vi "Core_Chem_User_Interface_v1.2.vi"() -> ()   [LabVIEW 2014]
uses:
  C:/Program Files (x86)/National Instruments/LabVIEW 2014/examples/Data Communication/Network Streams/Simple Network Streams/support/Network Stream Command.ctl
  <vilib>/dex/Stream Element Allocation Mode.ctl
  <vilib>/Platform/TimedLoop/XDataNode/timing_clust.ctl
  <vilib>/Platform/TimedLoop/XDataNode/nitl_modes.ctl
  <vilib>/Platform/TimedLoop/XDataNode/wakeup.ctl
  <vilib>/Utility/tcp.llb/UDP Multicast Read-Only Open.vi
  <vilib>/platform/TimedLoop/XDataNode/XDataNode.xnode
  <vilib>/Platform/TimedLoop/XDataNode/XDNodeRunTimeDep.lvlib
  <vilib>/FTP/NI_FTP.lvlib
panel:
  out "Create folder error out 2":errorcluster
  out "Network to cRIO live status":bool
  out "Create folder error out":errorcluster
  in  "Confirm Flight Number":bool
  out "PRTAFT_UDP_In":string
  out "TWBOZO01":string
  out "CABOZO01":string
  out "TEIOZO01":string
  out "CHTSOO01":string
  out "CHFGGA01":string
  out "AL52CO01":string
  in  "Flight Number":string
  in  "Tab Control":T1(tab)
  out "PRTAFT_DLU":string
  out "MFM":dbl(graph)
  in  "name":string="239.1.4.6"
  in  "Port":u16=50001
  out "FGGA":string
  out "CO":string
  out "Ozone":string
  out "Cabin Ozone":string
  out "Ambient Ozone":string
  out "SO2":string
  out "Raw Signal":dbl(graph)
  out "CO Concentration":dbl(graph)
  out "Fluorsecence Cell Pressure":dbl(graph)
  out "Monochromater Flow":dbl(graph)
  out "Lamp Flow Controller":dbl(graph)
  in  "CO UDP Time Offset":i32=1
  out "CO2 Pressure\nDelivery (PSIA)":dbl(slide) scale=0.0..100.0
  out "CO CAL Status":bool
  out "Std\nContent (barG)":dbl(slide) scale=0.0..220.0
  out "N2\nContent (barG)":dbl(slide) scale=0.0..220.0
  out "CO2\nContent (barG)":dbl(slide) scale=0.0..170.0
  in  "CO CAL":bool
  in  "CO Vacuum (eV7)":bool
  out "CO Event error out":errorcluster
  out "CO command sender error out":errorcluster
  out "CO Zero":T2(array[cluster])
  out "CO Sensitivity":T3(array[cluster])
  in  "Ozone eV6":bool
  out "TEI49C Sample Flow B":dbl(graph)
  out "TEi49C Concentration":dbl(graph)
  out "TEI49C Sample Flow A":dbl(graph)
  out "Ozone Event error out":errorcluster
  out "Ozone command sender error out":errorcluster
  out "Ozone Zeroing\nTime Remain (sec)":u32
  in  "Ozone Zeroing":bool
  in  "Ozone UDP Time Offset":i32=1
  in  "FGGA Pump":bool
  in  "FGGA Shutdown":bool
  in  "eV1":bool
  in  "eV2":bool
  in  "MFC_1\nSLPM Value":dbl
  in  "eV3":bool
  in  "eV4":bool
  in  "FGGA Restart":bool
  out "MFC1 Cal Flow":dbl(graph)
  out "Cell temperature":dbl(graph)
  out "Cell pressure":dbl(graph)
  out "CO2 Dry":dbl(graph)
  out "CH4 Dry":dbl(graph)
  out "H2O":dbl(graph)
  out "CO2":dbl(graph)
  out "CH4":dbl(graph)
  in  "Flush High Tank":bool
  in  "Flush Low Tank":bool
  in  "Flush Target Tank":bool
  out "Flush High Tank\nTime Remain (sec)":u32
  out "Flush Low Tank\nTime Remain (sec)":u32
  out "Flush Target Tank\nTime Remain (sec)":u32
  in  "High Cal":bool
  out "High Cal\nFlush Time Remain (sec)":u32
  out "High Cal\nCal Time Remain (sec)":u32
  in  "Low Cal":bool
  in  "Target Cal":bool
  in  "Span Cal":bool
  out "Low Cal\nFlush Time Remain (sec)":u32
  out "Low Cal\nCal Time Remain (sec)":u32
  out "Target Cal\nFlush Time Remain (sec)":u32
  out "Target Cal\nCal Time Remain (sec)":u32
  in  "MFC_1 User Set Value":dbl=3.0
  out "FGGA command sender error out":errorcluster
  out "FGGA Event Error out":errorcluster
  in  "FGGA UDP Time Offset":i32=1
  in  "FGGA pump\nsync to WoW":bool
  out "WoW Flag":string="0"
  in  "Inst_alm_thresh":i32=220
  in  "3hr_alm_thresh":i32=80
  in  "Simulate Inst Conc":i32
  in  "Simulate 3hr Average Conc":dbl
  in  "Simulate 2B Conc":bool
  out "2B Ozone concentration":dbl(graph)
  out "2B Ozone flow rate":dbl(graph)
  out "2BOzone Event error out":errorcluster
  out "2BOzone command sender error out":errorcluster
  in  "Ambient = OFF\nCabin = ON":bool
  in  "eV9 Flush User\nset time (sec)":i32=15
  in  "eV9 flush User\nset time (sec)":i32=60
  in  "eV8 User\nset time (sec)":i32=120
  in  "eV9":bool
  in  "eV8":bool
  in  "SO2 eV6":bool
  in  "MFC_2\nSLPM Value":dbl
  in  "MFC_3\nSLPM Value":dbl=2.0
  in  "Simulate STEL Conc":dbl
  in  "Simulate TWA Conc":dbl
  in  "SO2 Offset":dbl
  in  "SO2 Slope":dbl=1.0
  in  "10mins STEL Limit":i32=700
  in  "8hr TWA Limit":i32=490
  in  "Simulate Conc":bool
  out "TEI43i MFC2 Cal Flow":dbl(graph)
  out "TEI43i MFC3 Sample Flow":dbl(graph)
  out "TEi43C Concentration":dbl(graph)
  out "TEI43C Sample Flow":dbl(graph)
  out "SO2 Event error out":errorcluster
  out "SO2 command sender error out":errorcluster
  in  "SO2 Flush":bool
  in  "SO2 CAL":bool
  in  "MFC_2 User Set Value":dbl=2.5
  in  "MFC_3 User Set Value":dbl=2.0
  out "SO2 Flush\nTime Remain (sec)":u32
  in  "SO2 Zeroing":bool
  out "SO2 Zeroing\nTime Remain (sec)":u32
  out "SO2 CAL\nTime Remain (sec)":u32
  in  "SO2 UDP Time Offset":i32=1
  in  "cRIO File IO Stop\n(USB Flash Drive Unmount)":bool
  in  "FTP ASCII Files to Local":bool
  in  "Transfer FGGA Files":bool
  out "File List":string[](array[string])
  out "FGGA File Transfer Error out":errorcluster
  out "Move to FM Error out":errorcluster
  out "USB Disk Space Used %":dbl(slide) scale=0.0..100.0
  out "PTP Sync":bool
  out "CPU Total %":dbl(graph)
  # "ch4\nco2\nh2o\npress_torr\ntemp_c\nfit_flag\nrda_usec\nrdb_usec\nch4_dry\nco2_dry\nMFC_1_absolute_pressure\nMFC_1_temperature\nMFC_1volumetic_flow\nMFC_1mass_flow\nMFC_1set_point\nV1\nV2\nV3\nV4\nrestart_FGGA\nFGGA_Pump\nCAL_MFC_1Set_Value"
  # "conc\ntemp\npress\nflow\nthreehr_oz\nInst_alarm\nthreehr_alarm"
  # "conc\ntemp\npress\nflow"
  # "concentration\npmt_volt\nlamp_volt\nlamp_intens\ninternal_temper\nreact_temper\nreact_press\nflow\nflags\nten_min_so2\neight_hr_so2\nten_min_so2_alm\neight_hr_so2_alm\nMFC_2absolute_pressure\nMFC_2temperature\nMFC_2volumetic_flow\nMFC_2mass_flow\nMFC_2set_point\nMFC_3_absolute_pressure\nMFC_3_temperature\nMFC_3volumetic_flow\nMFC_3mass_flow\nMFC_3set_point\nV6\nV8\nV9\nMFC2_Set_Value\nMFC3_Set_Value"
  # "conc\nbenchtemp\npress\ncellAint\ncellBint\nFlowA\nFlowB\nlamptemp\nflag\nV6"
  # "conc\ncounts\nsens\nzero\nlampflow\nlamptemp\nmonoflow\nmonotemp\nmonopress\ncellpress\ncalpress\ntemppmt\ncalconc\nerr\ncal_counter\nerr_counter\nCO_vacuum_status\nIn_Cal\nALEG1_press_delivery\nALREG1_press_content\nALREG2_press_content\nALREG3_press_content"
  # "DIRECT CONTROL"
  # "DIRECT CONTROLS"
  # "DIRECT CONTROLS"
  # "TEi43c"
  # "TEi43i"
  # "SO2 FLUSH SETTING"
  # "SO2 CAL SETTINGS"
  # "DIRECT CONTROLS"
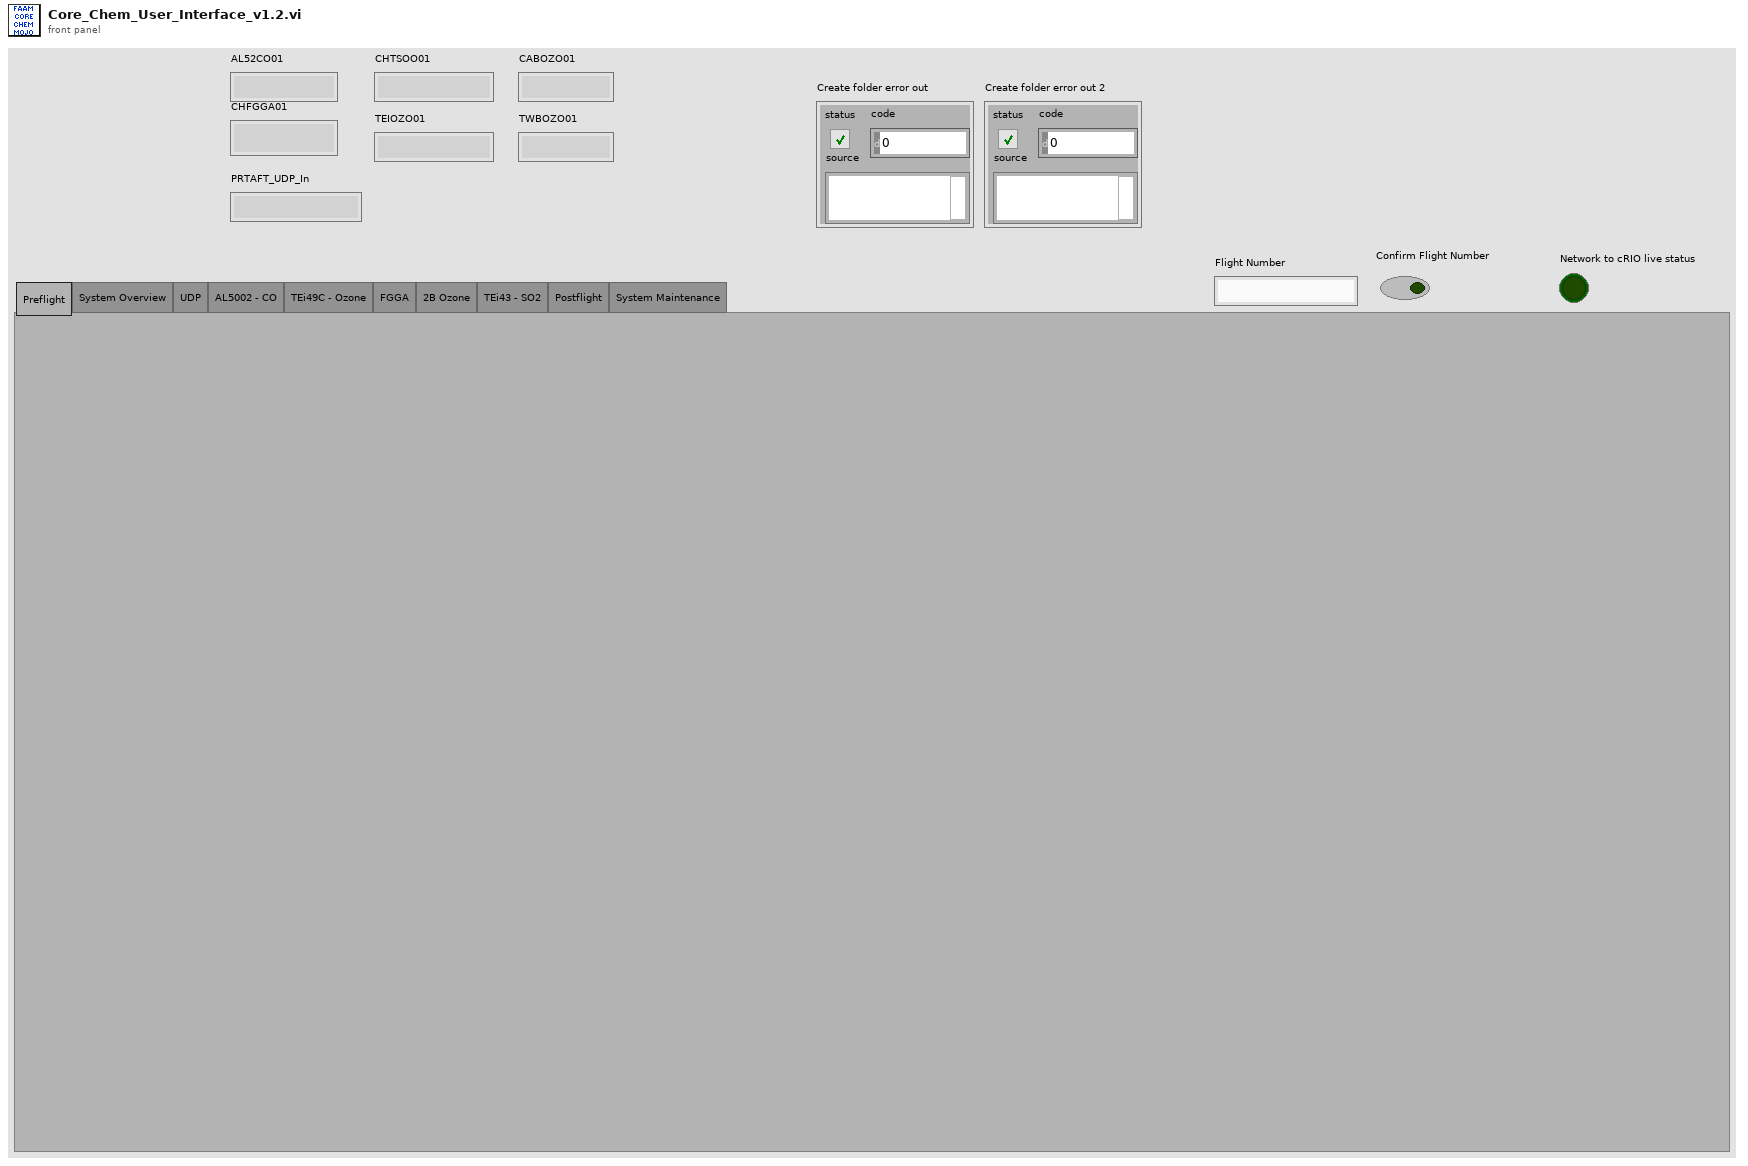
[diagram p1: front panel]
types:
  T1 = enum32{"Preflight", "System Overview", "UDP", "AL5002 - CO", "TEi49C - Ozone", "FGGA", "2B Ozone", "TEi43 - SO2", "Postflight", "System Maintenance"}
  T2 = cluster{"time stamp":timestamp, "CO Offset":dbl}[]
  T3 = cluster{"time stamp":timestamp, "CO Sensitivity":dbl}[]
  T4 = typedef "Network Stream Command.ctl" = cluster{"Message":string, "Message Data":variant}
  T5 = typedef "Stream Element Allocation Mode.ctl" = u32
  T6 = typedef "XDNodeRunTimeDep.lvlib/timing_clust.ctl" = cluster{"Expected End [f-1]":u64, "Actual End [f-1]":u64, "Finished Late? [f-1]":bool, "Expected End [i-1]":u64, "Actual End [i-1]":u64, "Finished Late? [i-1]":bool, "Expected Start [i]":u64, "Actual Start [i]":u64, "Expected Start [f]":u64, "Actual Start [f]":u64, "Source Name":string, "Structure Name":string, "Period":i64, "Deadline":i64, "Offset":i64, "Start":i64, "Priority":i32, "Timeout":i32, "Mode":T7, "Wakeup Reason":T8, "Error":errorcluster, "Source Type":string, "Secondary Source Type":string, "Global End Time":u64, "Global Start Time":u64, "Frame Duration":u64, "Iteration Duration":u64, "Assigned CPU":i32, "I/O Scan Engine Mode":u32}
  T7 = typedef "XDNodeRunTimeDep.lvlib/nitl_modes.ctl" = enum32{"No Change", "Process missed periods, maintain original phase", "Discard missed periods, maintain original phase", "Process missed periods, ignore original phase", "Discard missed periods, ignore original phase"}
  T8 = typedef "XDNodeRunTimeDep.lvlib/wakeup.ctl" = enum32{"Normal", "Aborted", "Asynchronous wakeup", "Timing source error", "Timed loop error", "Timeout"}
  T9 = typedef "NI_FTP.lvlib/FTP Session.ctl" = refnum<k5>
  T10 = typedef "NI_FTP.lvlib/FTP File Info.ctl" = cluster{"type":enum16{"unknown", "file", "dir", "link"}, "permissions":string, "owner":string, "group":string, "size":i32, "date":string, "name":string, "link name":string}
  T11 = cluster{"Message":string, "Message 2":string, "Message 3":string}
  T12 = cluster{"Message":string, "Message 2":string, "Message 3":string, "Message 4":string}
  T13 = cluster{"Message":string, "Message 3":string, "Message 4":string}
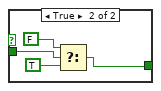
[diagram p8: hidden frame]
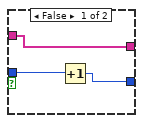
[diagram p13: hidden frame]
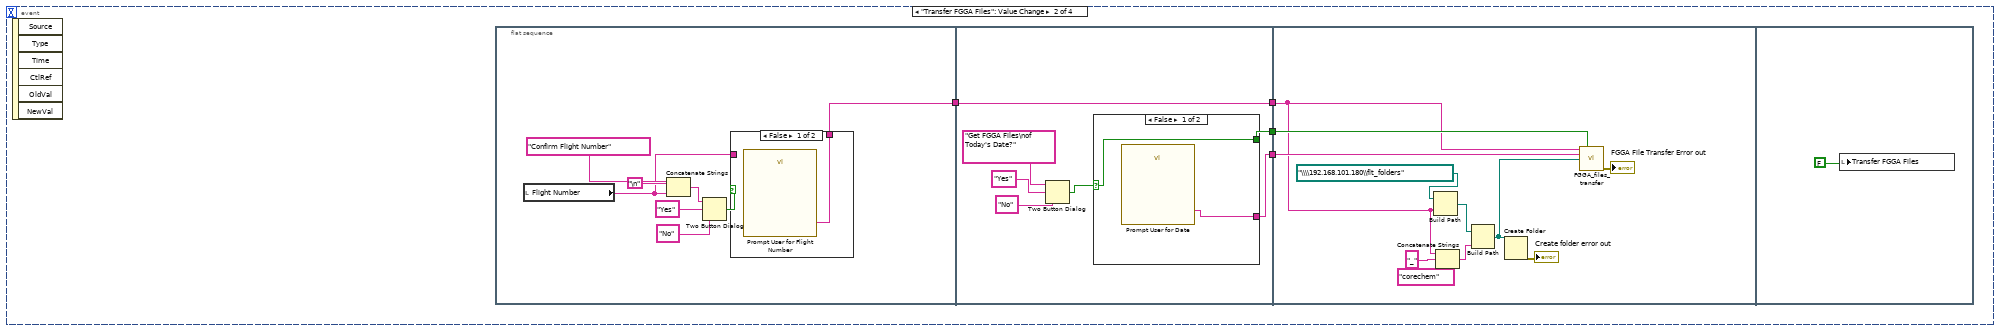
[diagram p15: hidden frame]
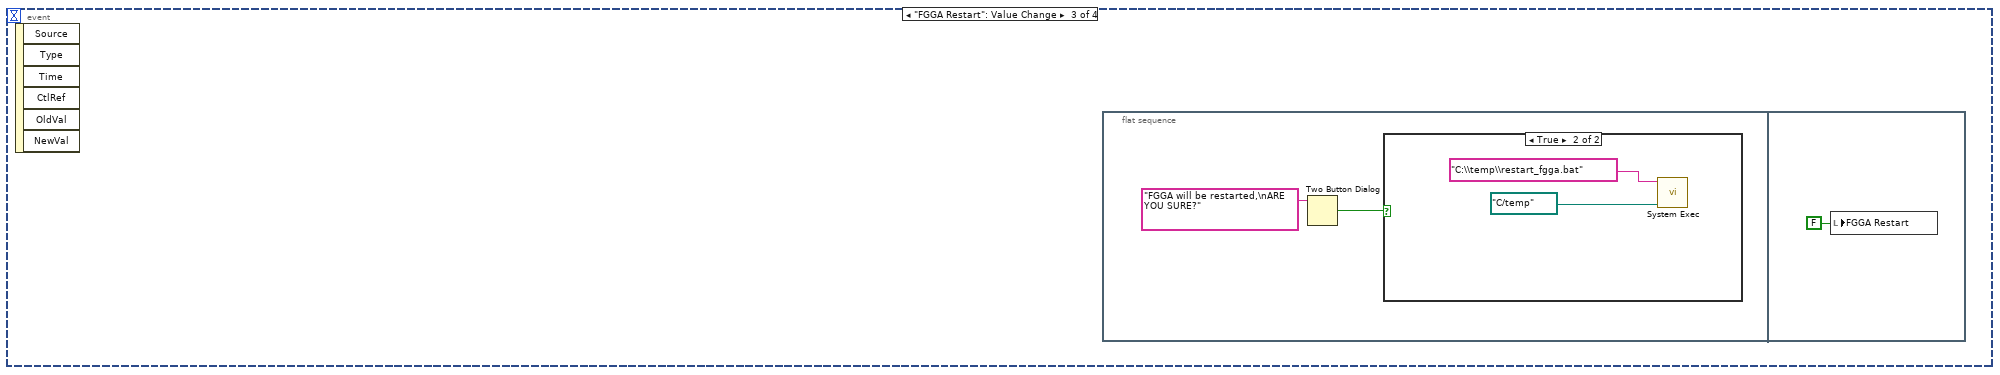
[diagram p18: hidden frame]
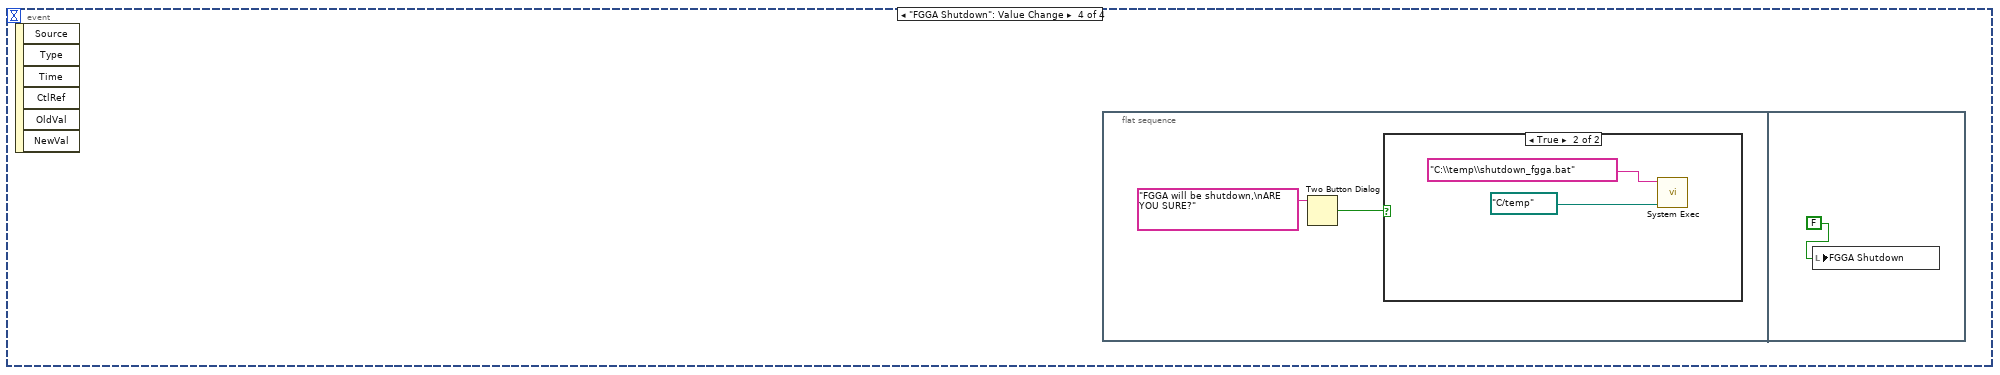
[diagram p20: hidden frame]
diagram:
  w4 = "XXXX"
  w7 = 0
  w8 = 0.0
  w14 = T4 {"Message"="", "Message Data"=variant} ("Message Cluster")
  w20 = T5 0 items=["allocate as needed", "pre-allocate"] ("element allocation mode")
  w26 = T4 {"Message"="", "Message Data"=variant} ("Message Cluster")
  w32 = T5 0 items=["allocate as needed", "pre-allocate"] ("element allocation mode")
  w37 = T4 {"Message"="", "Message Data"=variant} ("Message Cluster")
  w43 = T5 0 items=["allocate as needed", "pre-allocate"] ("element allocation mode")
  w53 = T5 0 items=["allocate as needed", "pre-allocate"] ("element allocation mode")
  w55 = T4 {"Message"="", "Message Data"=variant} ("Message Cluster")
  w62 = T5 0 items=["allocate as needed", "pre-allocate"] ("element allocation mode")
  w64 = T4 {"Message"="", "Message Data"=variant} ("Message Cluster")
  n1 = local write "cRIO File IO Stop\n(USB Flash Drive Unmount)"(FALSE ("Stop File Write")) -> ()
  n2 = local write "Flight Number"(w4) -> ()
  n3 = while {
    shift-right: [w68] -> _
    shift-left: w4 -> [w67]
    stop <- FALSE stop-if-true
    n4 = Not Equal?(x=w67, y="Flight Number") -> (x != y?=w70:bool)
    n5 = case shown="True" w70 {
      tunnel: [w73 w74] -> w68
      tunnel: "Flight Number" -> [_ w74]
      tunnel: w67 -> [w73 _]
      frame False {
      }
      frame True {
        n6 = One Button Dialog(message="Flight Number changed,\nPress flight number button to confirm") -> ()  [unwired: 1 in, 1 out]
      }
    }
    n7 = Wait (ms)(milliseconds to wait=u32 1000) -> ()  [unwired: 1 out]
  }
  n8 = while {
    stop <- FALSE stop-if-true
    # "UDP Read"
    n9 = String To IP(1:"name") -> (0:w81:u32)
    n10 = call-poly <vilib>:"UDP Multicast Open.vi"("multicast addr"=w81, "port"="Port") -> ("error out"=w79:errorcluster, "connection ID"=w78:refnum<k16>)  [unwired: 7 in, 1 out]
    n11 = Wait (ms)(milliseconds to wait=u32 1000) -> ()  [unwired: 1 out]
    n12 = case shown="No Error" w79 {
      selector: w79 -> [w85 _]
      tunnel: w78 -> [w84 _]
      frame No Error {
        w83 = ""
        n13 = while {
          tunnel: w85 -> [w131]
          tunnel: w84 -> [w130]
          shift-right: [w126] -> _
          shift-left: w83 -> [w127]
          shift-right: [w117] -> _
          shift-left: w83 -> [w119]
          shift-right: [w111] -> _
          shift-left: w83 -> [w113]
          shift-right: [w105] -> _
          shift-left: w83 -> [w106]
          shift-right: [w99] -> _
          shift-left: w83 -> [w100]
          shift-right: [w93] -> _
          shift-left: w83 -> [w94]
          shift-right: [w87] -> _
          shift-left: w83 -> [w88]
          stop <- w129 stop-if-true
          n14 = UDP Read(connection ID=w130, 8:w131) -> (data out=w86:string, error out=w129:errorcluster)  [unwired: 2 in, 3 out]
          n15 = Match Pattern(string=w86, regular expression="$TEIOZO01,") -> (match substring=w125:string, after substring=w124:string)  [unwired: 1 in, 2 out]
          n16 = Match Pattern(string=w86, regular expression="$TWBOZO01,") -> (match substring=w103:string, after substring=w102:string)  [unwired: 1 in, 2 out]
          n17 = Match Pattern(string=w86, regular expression="$CABOZO01,") -> (match substring=w109:string, after substring=w108:string)  [unwired: 1 in, 2 out]
          n18 = Match Pattern(string=w86, regular expression="$CHTSOO01,") -> (match substring=w97:string, after substring=w96:string)  [unwired: 1 in, 2 out]
          n19 = Match Pattern(string=w86, regular expression="$CHFGGA01,") -> (match substring=w121:string, after substring=w120:string)  [unwired: 1 in, 2 out]
          n20 = Match Pattern(string=w86, regular expression="$AL52CO01,") -> (match substring=w115:string, after substring=w114:string)  [unwired: 1 in, 2 out]
          n21 = Match Pattern(string=w86, regular expression="$PRTAFT01,") -> (match substring=w92:string, after substring=w91:string)  [unwired: 1 in, 2 out]
          n22 = Concatenate Strings(w125, w124) -> (w123:string)
          n23 = Concatenate Strings(w103, w102) -> (w101:string)
          n24 = Concatenate Strings(w109, w108) -> (w107:string)
          n25 = Concatenate Strings(w97, w96) -> (w95:string)
          n26 = Concatenate Strings(w121, w120) -> (w118:string)
          n27 = Concatenate Strings(w115, w114) -> (w112:string)
          n28 = Concatenate Strings(w92, w91) -> (w89:string)
          n29 = Replace Substring(4:w101, 5:w100) -> (1:w99:string)  [unwired: 2 in, 1 out]
          "TWBOZO01" <- w99
          n30 = Replace Substring(4:w123, 5:w127) -> (1:w126:string)  [unwired: 2 in, 1 out]
          "TEIOZO01" <- w126
          n31 = Replace Substring(4:w107, 5:w106) -> (1:w105:string)  [unwired: 2 in, 1 out]
          "CABOZO01" <- w105
          n32 = Replace Substring(4:w95, 5:w94) -> (1:w93:string)  [unwired: 2 in, 1 out]
          "CHTSOO01" <- w93
          n33 = Replace Substring(4:w112, 5:w113) -> (1:w111:string)  [unwired: 2 in, 1 out]
          "AL52CO01" <- w111
          n34 = Replace Substring(4:w118, 5:w119) -> (1:w117:string)  [unwired: 2 in, 1 out]
          "CHFGGA01" <- w117
          n35 = Replace Substring(4:w89, 5:w88) -> (1:w87:string)  [unwired: 2 in, 1 out]
          "PRTAFT_UDP_In" <- w87
        }
      }
      frame Error {
      }
    }
  }
  n36 = Obtain Queue(name (unnamed)="CO_Command", element data type=w64) -> (queue out=w13:refnum<queue>, error out=w58:errorcluster)  [unwired: 3 in, 1 out]
  n37 = Create Network Stream Writer Endpoint(6:w62, 7:10 ("writer buffer size"), 9:w64, 10:"//192.168.101.17/command/reader/CO" ("reader url"), 11:"/command/writer/CO" ("writer name")) -> (0:w61:errorcluster, 3:w60:refnum<k21>)  [unwired: 2 in]
  n38 = while {
    tunnel: w13 -> [w135]
    tunnel: w58 -> [w134]
    tunnel: [w132] -> _
    stop <- FALSE stop-if-true
    # "CO UI Event Handler Loop"
    n39 = event shown="[4] \"Confirm Flight Number\": Value Change" {
      selector: _ -> [_ _ _ _ _]
      dyn-events: _ -> [_ _ _ _ _]
      timeout: _ -> [_ _ _ _ _]
      tunnel: w135 -> [w142 w149 w153 w160 w167]
      tunnel: w134 -> [w141 w148 w152 w159 w166]
      tunnel: [w136 w143 w151 w158 w165] -> w132
      event "CO CAL": Value Change {
        n40 = event-data() -> ("NewVal"=w139:bool)  [unwired: 1 in]
        n41 = Bundle(cluster=T4 {"Message"="", "Message Data"=variant} ("Message Cluster"), "Message"="CO CAL", "Message Data"=w139) -> (w137:T4)
        n42 = Enqueue Element(queue=w142, element=w137, error in (no error)=w141) -> (error out=w136:errorcluster)  [unwired: 1 in, 2 out]
      }
      event "CO UDP Time Offset": Value Change {
        n43 = event-data() -> ("NewVal"=w146:i32)  [unwired: 1 in]
        n44 = Bundle(cluster=T4 {"Message"="", "Message Data"=variant} ("Message Cluster"), "Message"="UDP Time Offset", "Message Data"=w146) -> (w144:T4)
        n45 = Enqueue Element(queue=w149, element=w144, error in (no error)=w148) -> (error out=w143:errorcluster)  [unwired: 1 in, 2 out]
      }
      event "CO Vacuum (eV7)": Value Change {
        n46 = event-data() -> ("NewVal"=w150:bool)  [unwired: 1 in]
        n47 = Bundle(cluster=T4 {"Message"="", "Message Data"=variant} ("Message Cluster"), "Message"="CO Vacuum", "Message Data"=w150) -> (w154:T4)
        n48 = Enqueue Element(queue=w153, element=w154, error in (no error)=w152) -> (error out=w151:errorcluster)  [unwired: 1 in, 2 out]
      }
      event "cRIO File IO Stop\n(USB Flash Drive Unmount)": Value Change {
        n49 = event-data() -> ("NewVal"=w157:bool)  [unwired: 1 in]
        n50 = Bundle(cluster=T4 {"Message"="", "Message Data"=variant} ("Message Cluster"), "Message"="Stop File Write", "Message Data"=w157) -> (w161:T4)
        n51 = Enqueue Element(queue=w160, element=w161, error in (no error)=w159) -> (error out=w158:errorcluster)  [unwired: 1 in, 2 out]
      }
      event "Confirm Flight Number": Value Change {
        n52 = event-data() -> ()  [unwired: 1 in, 1 out]
        n53 = local read "Flight Number"() -> (w164:string)
        n54 = Bundle(cluster=T4 {"Message"="", "Message Data"=variant} ("Message Cluster"), "Message"="Flight Number", "Message Data"=w164) -> (w168:T4)
        n55 = Enqueue Element(queue=w167, element=w168, error in (no error)=w166) -> (error out=w165:errorcluster)  [unwired: 1 in, 2 out]
      }
    }
    "CO Event error out" <- w132
  }
  n56 = while {
    tunnel: w13 -> [w178]
    shift-right: [w173] -> _
    shift-left: w60 -> [w175]
    shift-right: [w171] -> w49
    shift-left: w61 -> [w177]
    tunnel: w58 -> [w172]
    stop <- w171 stop-if-true
    # "CO UI Command Sender"
    n57 = Dequeue Element(queue=w178, error in (no error)=w172) -> (element=w174:T4)  [unwired: 1 in, 3 out]
    n58 = Unbundle By Name(w174) -> ("Message"=w176:string)
    n59 = case shown="\"UDP Time Offset\"" w176 {
      tunnel: w177 -> [w179 w183 w190 w197 w204 w211]
      tunnel: w175 -> [w180 w186 w193 w200 w207 w214]
      tunnel: w174 -> [_ w185 w192 w199 w206 w213]
      tunnel: [w179 w182 w189 w196 w203 w210] -> w171
      tunnel: [w180 w181 w188 w195 w202 w209] -> w173
      frame "False", Default {
      }
      frame "CO CAL" {
        n60 = shared-variable-write(w186, w183, w185) -> (w184:refnum<k21>, w187:errorcluster)  [unwired: 1 in, 1 out]
        n61 = Flush Stream(8:w187, 11:w184) -> (0:w182:errorcluster, 3:w181:refnum<k21>)  [unwired: 2 in, 1 out]
      }
      frame "UDP Time Offset" {
        n62 = shared-variable-write(w193, w190, w192) -> (w191:refnum<k21>, w194:errorcluster)  [unwired: 1 in, 1 out]
        n63 = Flush Stream(8:w194, 11:w191) -> (0:w189:errorcluster, 3:w188:refnum<k21>)  [unwired: 2 in, 1 out]
      }
      frame "Stop File Write" {
        n64 = shared-variable-write(w200, w197, w199) -> (w198:refnum<k21>, w201:errorcluster)  [unwired: 1 in, 1 out]
        n65 = Flush Stream(8:w201, 11:w198) -> (0:w196:errorcluster, 3:w195:refnum<k21>)  [unwired: 2 in, 1 out]
      }
      frame "Flight Number" {
        n66 = shared-variable-write(w207, w204, w206) -> (w205:refnum<k21>, w208:errorcluster)  [unwired: 1 in, 1 out]
        n67 = Flush Stream(8:w208, 11:w205) -> (0:w203:errorcluster, 3:w202:refnum<k21>)  [unwired: 2 in, 1 out]
      }
      frame "CO Vacuum" {
        n68 = shared-variable-write(w214, w211, w213) -> (w212:refnum<k21>, w215:errorcluster)  [unwired: 1 in, 1 out]
        n69 = Flush Stream(8:w215, 11:w212) -> (0:w210:errorcluster, 3:w209:refnum<k21>)  [unwired: 2 in, 1 out]
      }
    }
  }
  "CO command sender error out" <- w49
  n70 = node-c288() -> (w12:T6)  [unwired: 4 in]
  n71 = Initialize Array(cluster{"time stamp":timestamp, "Y":dbl} {"time stamp"=timestamp(0 s since 1904-01-01), "Y"=0.0}, 30 ("dimension size")) -> (w9:cluster{"time stamp":timestamp, "Y":dbl}[])
  n72 = timed-loop {
    timing: w12 -> [_]
    timing-out: [_] -> w11
    stop <- _ stop-if-true
    # "PC Tasks"
    n73 = node-c288() -> ()  [unwired: 1 in, 1 out]
    n74 = event shown="[0] \"FTP ASCII Files to Local\": Value Change" {
      selector: _ -> [_ _ _ _]
      dyn-events: _ -> [_ _ _ _]
      timeout: _ -> [_ _ _ _]
      event "FTP ASCII Files to Local": Value Change {
        n75 = event-data() -> ()  [unwired: 1 in, 1 out]
        n76 = flat-sequence {
          tunnel: [w224] -> w218
          tunnel: [w236] -> w223
          tunnel: [w235] -> w221
          tunnel: [w234] -> w219
          tunnel: w218 -> [w234]
          tunnel: w223 -> [w294]
          tunnel: [w294] -> w222
          tunnel: w221 -> [w290]
          tunnel: [w289] -> w220
          tunnel: w219 -> [w289]
          tunnel: w222 -> [w300]
          tunnel: w220 -> [w295]
          frame #0 {
            n77 = local read "Flight Number"() -> (w226:string)
            n78 = Concatenate Strings("Confirm Flight Number" ("message"), "\n", w226) -> (w230:string)
            n79 = Two Button Dialog(message=w230, 1:"No" ("F button name (\"Cancel\")"), 2:"Yes" ("T button name (\"OK\")")) -> (T button?=w227:bool)
            n80 = case shown="False" w227 {
              tunnel: w226 -> [_ w233]
              tunnel: [w232 w233] -> w224
              frame False {
                n81 = call "Prompt User for Flight Number2"() -> ("Flight Number BXXX"=w232:string)  [unwired: 17 in, 2 out]
              }
              frame True {
              }
            }
          }
          frame #1 {
            n82 = Get Date/Time In Seconds() -> (seconds since 1Jan1904=w240:timestamp)
            n83 = Format Date/Time String(time format string (%c)="%Y%m%d", seconds (now)=w240) -> (date/time string=w238:string)  [unwired: 1 in]
            n84 = call <vilib>:"FTP Open Session.vi"("address"="192.168.101.17") -> ("error out"=w255:errorcluster, "ftp session"=w256:T9)  [unwired: 7 in, 2 out]
            n85 = Concatenate Strings("Use Today's Date" ("message"), "\r", w238) -> (w244:string)
            n86 = call <vilib>:"FTP Logon.vi"("error in (no error)"=w255, "password"="", "user"="anonymous", "ftp session"=w256) -> ("error out"=w252:errorcluster, "ftp session out"=w251:T9)  [unwired: 4 in, 2 out]
            n87 = Two Button Dialog(message=w244, 1:"No" ("F button name (\"Cancel\")"), 2:"Yes" ("T button name (\"OK\")")) -> (T button?=w241:bool)
            n88 = case shown="False" w241 {
              tunnel: [w259 w260] -> w235
              tunnel: w238 -> [_ w260]
              frame False {
                n89 = call "Prompt User for Date"() -> ("Date"=w259:string)  [unwired: 17 in, 2 out]
              }
              frame True {
              }
            }
            n90 = call <vilib>:"FTP Directory Listing.vi"("error in (no error)"=w252, "directory path"="/U:/data", "ftp session"=w251) -> ("dir list"=w250:T10[])  [unwired: 4 in, 4 out]
            n91 = for {
              tunnel: w250 -> [w280] mode=indexing
              tunnel: [w279] -> w247 mode=indexing
              tunnel: w235 -> [w278]
              # "Extract File Name According to the Date"
              n92 = Unbundle By Name(w280) -> ("name"=w286:string, "name"=w285:string)
              n93 = Match Pattern(string=w285, regular expression="_[0-9]+") -> (match substring=w283:string)  [unwired: 1 in, 3 out]
              n94 = String Subset(string=w283, offset (0)=1) -> (substring=w281:string)  [unwired: 1 in]
              n95 = Equal?(x=w281, y=w278) -> (x = y?=w287:bool)
              n96 = case shown="False" w287 {
                tunnel: w286 -> [_ w288]
                tunnel: [_ w288] -> w279
                frame False {
                }
                frame True {
                }
              }
            }
            n97 = Array Size(array=w247) -> (size(s)=w249:i32)
            n98 = for {
              N: w249 -> [_]
              shift-right: [w267] -> w237
              shift-left: w247 -> [w268]
              shift-right: [w265] -> _
              shift-left: 0 -> [w266]
              # "Remove Empty Array"
              n99 = Index Array(array=w268, index=w266) -> (element=w270:string)
              n100 = Equal?(x=w270, y="") -> (x = y?=w269:bool)
              n101 = case shown="True" w269 {
                tunnel: w268 -> [w274 w277]
                tunnel: w266 -> [w273 w275]
                tunnel: [w274 w276] -> w267
                tunnel: [w272 w275] -> w265
                frame False {
                  n102 = Increment(x=w273) -> (x+1=w272:i32)
                }
                frame True {
                  n103 = Delete From Array(array=w277, index=w275) -> (array with subset deleted=w276:string[])  [unwired: 1 in, 1 out]
                }
              }
            }
            "File List" <- w237
            n104 = for {
              tunnel: w237 -> [w263] mode=indexing
              tunnel: [w261] -> w236 mode=indexing
              # "Specify destination path for each file"
              n105 = Concatenate Strings("C:\\temp\\", w263) -> (w262:string)
              n106 = String To Path(string=w262) -> (path=w261:path)
            }
          }
          frame #2 {
            # "FTP a list of files"
            n107 = call <vilib>:"System Exec.vi"("wait until completion? (T)"=TRUE, "working directory"=path "C:/temp", "standard input"=w290, "command line"="C:\\temp\\transfer_ascii_files.bat") -> ()  [unwired: 4 in, 4 out]
          }
          frame #3 {
            # "Move file from local PC to Flight Folder"
            n108 = Build Path(base path=path "\\\\192.168.101.180\\flt_folders" ("path"), name or relative path=w295) -> (appended path=w302:path)
            n109 = Concatenate Strings(w295, "_" ("string"), "corechem" ("string")) -> (w301:string)
            n110 = Build Path(base path=w302, name or relative path=w301) -> (appended path=w297:path)
            n111 = Create Folder(path (use dialog)=w297) -> (created path=w296:path, error out=→"Create folder error out 2":errorcluster)  [unwired: 2 in, 1 out]
            n112 = for {
              tunnel: w296 -> [w309]
              tunnel: [w308] -> w299
              tunnel: w300 -> [w306] mode=indexing
              n113 = Copy(9:TRUE ("overwrite (F)"), 10:w309, 11:w306) -> (0:w308:errorcluster)  [unwired: 2 in, 2 out]
            }
            "Move to FM Error out" <- w299
          }
          frame #4 {
            n114 = local write "FTP ASCII Files to Local"(FALSE ("FTP Files to Local")) -> ()
          }
        }
      }
      event "Transfer FGGA Files": Value Change {
        n115 = event-data() -> ()  [unwired: 1 in, 6 out]
        n116 = flat-sequence {
          tunnel: [w315] -> w314
          tunnel: w314 -> [w327]
          tunnel: [w327] -> w313
          tunnel: [w326] -> w312
          tunnel: [w325] -> w311
          tunnel: w313 -> [w343]
          tunnel: w312 -> [w345]
          tunnel: w311 -> [w344]
          frame #0 {
            n117 = local read "Flight Number"() -> (w316:string)
            n118 = Concatenate Strings("Confirm Flight Number" ("message"), "\n", w316) -> (w318:string)
            n119 = Two Button Dialog(message=w318, 1:"No" ("F button name (\"Cancel\")"), 2:"Yes" ("T button name (\"OK\")")) -> (T button?=w322:bool)
            n120 = case shown="False" w322 {
              tunnel: w316 -> [_ w324]
              tunnel: [w323 w324] -> w315
              frame False {
                n121 = call "Prompt User for Flight Number"() -> ("Flight Number BXXX"=w323:string)  [unwired: 17 in, 2 out]
              }
              frame True {
              }
            }
          }
          frame #1 {
            n122 = Two Button Dialog(message="Get FGGA Files\nof Today's Date?", 1:"No" ("F button name (\"Cancel\")"), 2:"Yes" ("T button name (\"OK\")")) -> (T button?=w331:bool)
            n123 = case shown="False" w331 {
              selector: w331 -> [w333 w334]
              tunnel: [w333 w334] -> w325
              tunnel: [w332 _] -> w326
              frame False {
                n124 = call "Prompt User for Date"() -> ("Date"=w332:string)  [unwired: 17 in, 2 out]
              }
              frame True {
              }
            }
          }
          frame #2 {
            n125 = Build Path(base path=path "\\\\192.168.101.180\\flt_folders" ("path"), name or relative path=w343) -> (appended path=w337:path)
            n126 = Concatenate Strings(w343, "_" ("string"), "corechem" ("string")) -> (w336:string)
            n127 = Build Path(base path=w337, name or relative path=w336) -> (appended path=w342:path)
            n128 = Create Folder(path (use dialog)=w342) -> (error out=→"Create folder error out":errorcluster)  [unwired: 2 in, 2 out]
            n129 = call "FGGA_files_transfer.vi"("Flight_num"=w343, "Get current?"=w344, "Date"=w345, "Flight Folder Path"=w342) -> ("error IO"=→"FGGA File Transfer Error out":errorcluster)  [unwired: 11 in]
          }
          frame #3 {
            n130 = local write "Transfer FGGA Files"(FALSE) -> ()
          }
        }
      }
      event "FGGA Restart": Value Change {
        n131 = event-data() -> ()  [unwired: 1 in, 6 out]
        n132 = flat-sequence {
          frame #0 {
            n133 = Two Button Dialog(message="FGGA will be restarted,\nARE YOU SURE?") -> (T button?=w348:bool)  [unwired: 2 in]
            n134 = case shown="True" w348 {
              frame False {
              }
              frame True {
                n135 = call <vilib>:"System Exec.vi"("working directory"=path "C:/temp", "command line"="C:\\temp\\restart_fgga.bat") -> ()  [unwired: 6 in, 4 out]
              }
            }
          }
          frame #1 {
            n136 = local write "FGGA Restart"(FALSE ("FGGA Restart")) -> ()
          }
        }
      }
      event "FGGA Shutdown": Value Change {
        n137 = event-data() -> ()  [unwired: 1 in, 6 out]
        n138 = flat-sequence {
          frame #0 {
            n139 = Two Button Dialog(message="FGGA will be shutdown,\nARE YOU SURE?") -> (T button?=w353:bool)  [unwired: 2 in]
            n140 = case shown="True" w353 {
              frame False {
              }
              frame True {
                n141 = call <vilib>:"System Exec.vi"("working directory"=path "C:/temp", "command line"="C:\\temp\\shutdown_fgga.bat") -> ()  [unwired: 6 in, 4 out]
              }
            }
          }
          frame #1 {
            n142 = local write "FGGA Shutdown"(FALSE ("FGGA Restart")) -> ()
          }
        }
      }
    }
    n143 = node-c288() -> ()  [unwired: 1 in, 1 out]
  }
  n144 = while {
    shift-right: [w440] -> _
    shift-left: w8 -> [w438]
    shift-right: [w442] -> _
    shift-left: w7 -> [w443]
    shift-right: [w441] -> _
    shift-left: w9 -> [w445]
    shift-right: [w433] -> _
    shift-left: w9 -> [w435]
    shift-right: [w430] -> _
    shift-left: w8 -> [w429]
    shift-right: [w432] -> _
    shift-left: w7 -> [w434]
    shift-right: [w425] -> _
    shift-left: FALSE -> [w426]
    stop <- FALSE stop-if-true
    w372 = ""
    w367 = "%s" ("format string")
    w564 = "%s" ("format string")
    w569 = "%s" ("format string")
    w574 = "%s" ("format string")
    w580 = "%s" ("format string")
    w586 = "%s" ("format string")
    w590 = "%s" ("format string")
    # "UDP Data Processing"
    n145 = local read "CHFGGA01"() -> (w593:string)
    n146 = local read "TWBOZO01"() -> (w568:string)
    n147 = local read "AL52CO01"() -> (w585:string)
    n148 = local read "CABOZO01"() -> (w573:string)
    n149 = local read "TEIOZO01"() -> (w579:string)
    n150 = local read "CHTSOO01"() -> (w563:string)
    n151 = local read "PRTAFT_UDP_In"() -> (w365:string)
    n152 = local read "Ambient = OFF\nCabin = ON"() -> (w467:bool)
    n153 = Spreadsheet String To Array(delimiter (Tab)=",", format string=w590, spreadsheet string=w593, array type (2D Dbl)=string[] []) -> (array=w540:string[])
    n154 = Spreadsheet String To Array(delimiter (Tab)=",", format string=w586, spreadsheet string=w585, array type (2D Dbl)=string[] []) -> (array=w561:string[])
    n155 = Spreadsheet String To Array(delimiter (Tab)=",", format string=w574, spreadsheet string=w573, array type (2D Dbl)=string[] []) -> (array=w464:string[])
    n156 = Spreadsheet String To Array(delimiter (Tab)=",", format string=w580, spreadsheet string=w579, array type (2D Dbl)=string[] []) -> (array=w538:string[])
    n157 = Spreadsheet String To Array(delimiter (Tab)=",", format string=w569, spreadsheet string=w568, array type (2D Dbl)=string[] []) -> (array=w463:string[])
    n158 = Spreadsheet String To Array(delimiter (Tab)=",", format string=w564, spreadsheet string=w563, array type (2D Dbl)=string[] []) -> (array=w536:string[])
    n159 = Array To Spreadsheet String(delimiter (Tab)="\r", array=w540, 3:w590) -> (spreadsheet string=→"FGGA":string)
    n160 = Array To Spreadsheet String(delimiter (Tab)="\r", array=w561, 3:w586) -> (spreadsheet string=→"CO":string)
    n161 = Array To Spreadsheet String(delimiter (Tab)="\r", array=w464, 3:w574) -> (spreadsheet string=→"Cabin Ozone":string)
    n162 = Array To Spreadsheet String(delimiter (Tab)="\r", array=w538, 3:w580) -> (spreadsheet string=→"Ozone":string)
    n163 = Spreadsheet String To Array(delimiter (Tab)=",", format string=w367, spreadsheet string=w365, array type (2D Dbl)=string[] []) -> (array=w366:string[])
    n164 = Array To Spreadsheet String(delimiter (Tab)="\r", array=w463, 3:w569) -> (spreadsheet string=→"Ambient Ozone":string)
    n165 = Array To Spreadsheet String(delimiter (Tab)="\r", array=w536, 3:w564) -> (spreadsheet string=→"SO2":string)
    n166 = Array To Spreadsheet String(delimiter (Tab)="\r", array=w366, 3:w367) -> (spreadsheet string=→"PRTAFT_DLU":string)
    n167 = Index Array(array=w366, index #1=5 ("index"), index #2=19 ("index")) -> (element #1=w370:string, element #2=w368:string)
    n168 = Select(t=w464, s=w467, f=w463) -> (s? t:f=w462:string[])
    n169 = Not Equal?(x=w370, y=w372) -> (x != y?=w371:bool)
    n170 = Not Equal?(x=w368, y=w372) -> (x != y?=w369:bool)
    n171 = Index Array(array=w536, index #1=6 ("index"), index #2=4 ("index"), index #3=3 ("index"), index #4=7 ("index"), index #5=8 ("index"), index #6=15 ("index"), index #7=24 ("index"), index #8=29 ("index")) -> (element #1=w453:string, element #2=w519:string, element #3=w514:string, element #4=w507:string, element #5=w483:string, element #6=w482:string, element #7=w390:string, element #8=w389:string)
    n172 = Index Array(array=w462, index #1=8 ("index"), index #2=11 ("index")) -> (element #1=w456:string, element #2=w457:string)
    n173 = Index Array(array=w538, index #1=6 ("index"), index #2=4 ("index"), index #3=3 ("index"), index #4=7 ("index"), index #5=9 ("index"), index #6=14 ("index"), index #7=15 ("index")) -> (element #1=w532:string, element #2=w520:string, element #3=w515:string, element #4=w500:string, element #5=w473:string, element #6=w472:string, element #7=w471:string)
    n174 = case shown="False" w369 {
      tunnel: ["1" w599] -> w362
      tunnel: w368 -> [_ w599]
      frame False {
      }
      frame True {
      }
    }
    n175 = case shown="False" w371 {
      tunnel: ["XXXX" w601] -> w363
      tunnel: w370 -> [_ w601]
      frame False {
      }
      frame True {
      }
    }
    n176 = Scan Value(string=w456, format string="%f") -> (value=→"2B Ozone concentration":dbl)  [unwired: 1 in, 1 out]
    n177 = Scan Value(string=w457, format string="%f") -> (value=→"2B Ozone flow rate":dbl)  [unwired: 1 in, 1 out]
    n178 = Scan Value(string=w390, format string="%f") -> (value=→"TEI43i MFC2 Cal Flow":dbl)  [unwired: 1 in, 1 out]
    n179 = Scan Value(string=w389, format string="%f") -> (value=→"TEI43i MFC3 Sample Flow":dbl)  [unwired: 1 in, 1 out]
    n180 = Scan Value(string=w483, format string="%f") -> (value=→"TEi43C Concentration":dbl)  [unwired: 1 in, 1 out]
    n181 = Scan Value(string=w482, format string="%f") -> (value=→"TEI43C Sample Flow":dbl)  [unwired: 1 in, 1 out]
    n182 = Index Array(array=w540, index #1=6 ("index"), index #2=4 ("index"), index #3=3 ("index"), index #4=7 ("index"), index #5=8 ("index"), index #6=9 ("index"), index #7=10 ("index"), index #8=17 ("index"), index #9=16 ("index"), index #10=11 ("index"), index #11=12 ("index"), index #12=21 ("index")) -> (element #1=w534:string, element #2=w522:string, element #3=w517:string, element #4=w502:string, element #5=w414:string, element #6=w411:string, element #7=w406:string, element #8=w404:string, element #9=w401:string, element #10=w396:string, element #11=w395:string, element #12=w382:string)
    n183 = local write "WoW Flag"(w362) -> ()
    n184 = local write "Flight Number"(w363) -> ()
    n185 = Index Array(array=w561, index #1=2 ("index"), index #2=27 ("index"), index #3=28 ("index"), index #4=29 ("index"), index #5=30 ("index"), index #6=31 ("index"), index #7=6 ("index"), index #8=4 ("index"), index #9=3 ("index"), index #10=8 ("index"), index #11=14 ("index"), index #12=16 ("index"), index #13=19 ("index"), index #14=12 ("index"), index #15=13 ("index"), index #16=10 ("index"), index #17=11 ("index")) -> (element #1=w424:string, element #2=w504:string, element #3=w551:string, element #4=w545:string, element #5=w543:string, element #6=w544:string, element #7=w533:string, element #8=w521:string, element #9=w516:string, element #10=w505:string, element #11=w492:string, element #12=w489:string, element #13=w488:string, element #14=w448:string, element #15=w447:string, element #16=w378:string, element #17=w359:string)
    n186 = Decimal String To Number(string=w424) -> (number=w422:i32)  [unwired: 2 in, 1 out]
    n187 = call "Find_Data_SubVI.vi"("FGGA"=w534, "CO"=w533, "Ozone"=w532, "SO2"=w453) -> ("Output Value"=→"CPU Total %":dbl)  [unwired: 11 in]
    n188 = call "Find_Data_SubVI.vi"("FGGA"=w522, "CO"=w521, "Ozone"=w520, "SO2"=w519) -> ("Output Value"=→"MFM":dbl)  [unwired: 11 in]
    n189 = call "Find_Data_SubVI.vi"("FGGA"=w517, "CO"=w516, "Ozone"=w515, "SO2"=w514) -> ("Output Value"=w513:dbl)  [unwired: 11 in]
    n190 = call "Find_Data_SubVI.vi"("FGGA"=w502, "CO"=w505, "Ozone"=w500, "SO2"=w507) -> ("Output Value"=→"USB Disk Space Used %":dbl)  [unwired: 11 in]
    n191 = Not Equal To 0?(x=w513) -> (x != 0?=→"PTP Sync":bool)
    n192 = Add(x=w422, y=u32 2082844800) -> (x+y=w421:u32)
    n193 = Scan Value(string=w382, format string="%f") -> (value=→"MFC1 Cal Flow":dbl)  [unwired: 1 in, 1 out]
    n194 = Scan Value(string=w395, format string="%f") -> (value=→"Cell temperature":dbl)  [unwired: 1 in, 1 out]
    n195 = Scan Value(string=w396, format string="%f") -> (value=→"Cell pressure":dbl)  [unwired: 1 in, 1 out]
    n196 = Scan Value(string=w401, format string="%f") -> (value=→"CH4 Dry":dbl)  [unwired: 1 in, 1 out]
    n197 = Scan Value(string=w404, format string="%f") -> (value=→"CO2 Dry":dbl)  [unwired: 1 in, 1 out]
    n198 = Scan Value(string=w406, format string="%f") -> (value=→"H2O":dbl)  [unwired: 1 in, 1 out]
    n199 = Scan Value(string=w411, format string="%f") -> (value=→"CO2":dbl)  [unwired: 1 in, 1 out]
    n200 = Scan Value(string=w414, format string="%f") -> (value=→"CH4":dbl)  [unwired: 1 in, 1 out]
    n201 = Scan Value(string=w544, format string="%f") -> (value=→"Std\nContent (barG)":dbl)  [unwired: 1 in, 1 out]
    n202 = Scan Value(string=w504, format string="%d", default (0 dbl)=u32 0) -> (value=w558:u32)  [unwired: 1 out]
    n203 = Scan Value(string=w543, format string="%f") -> (value=→"N2\nContent (barG)":dbl)  [unwired: 1 in, 1 out]
    n204 = Scan Value(string=w545, format string="%f") -> (value=→"CO2\nContent (barG)":dbl)  [unwired: 1 in, 1 out]
    n205 = Scan Value(string=w551, format string="%f") -> (value=→"CO2 Pressure\nDelivery (PSIA)":dbl)  [unwired: 1 in, 1 out]
    n206 = To Time Stamp(1:w421) -> (0:w428:timestamp)
    n207 = Scan Value(string=w473, format string="%f") -> (value=→"TEi49C Concentration":dbl)  [unwired: 1 in, 1 out]
    n208 = Scan Value(string=w472, format string="%f") -> (value=→"TEI49C Sample Flow A":dbl)  [unwired: 1 in, 1 out]
    n209 = Scan Value(string=w492, format string="%f") -> (value=→"Lamp Flow Controller":dbl)  [unwired: 1 in, 1 out]
    n210 = Scan Value(string=w359, format string="%f") -> (value=→"Raw Signal":dbl)  [unwired: 1 in, 1 out]
    n211 = Scan Value(string=w378, format string="%f") -> (value=→"CO Concentration":dbl)  [unwired: 1 in, 1 out]
    n212 = Scan Value(string=w471, format string="%f") -> (value=→"TEI49C Sample Flow B":dbl)  [unwired: 1 in, 1 out]
    n213 = Scan Value(string=w489, format string="%f") -> (value=→"Monochromater Flow":dbl)  [unwired: 1 in, 1 out]
    n214 = Scan Value(string=w488, format string="%f") -> (value=→"Fluorsecence Cell Pressure":dbl)  [unwired: 1 in, 1 out]
    n215 = Not Equal To 0?(x=w558) -> (x != 0?=→"CO CAL Status":bool)
    n216 = call "ping.vi"("Host IP Address"="192.168.101.17") -> ("connected?"=w427:bool)  [unwired: 14 in]
    n217 = Scan Value(string=w448, format string="%f") -> (value=w439:dbl)  [unwired: 1 in, 1 out]
    n218 = Scan Value(string=w447, format string="%f") -> (value=w431:dbl)  [unwired: 1 in, 1 out]
    n219 = Not Equal?(x=w438, y=w439) -> (x != y?=w444:bool)
    n220 = Not Equal?(x=w429, y=w431) -> (x != y?=w436:bool)
    n221 = case shown="True" w444 {
      tunnel: w445 -> [w619 w628]
      tunnel: w443 -> [w620 w627]
      tunnel: [w620 w626] -> w442
      tunnel: w428 -> [_ w622]
      tunnel: w439 -> [_ w623]
      tunnel: [w619 w625] -> w441
      tunnel: [w618 w624] -> w440
      tunnel: w439 -> [_ w624]
      tunnel: w438 -> [w618 _]
      frame False {
      }
      frame True {
        n222 = Bundle(w622, w623) -> (w621:cluster{timestamp, dbl})  [unwired: 1 in]
        n223 = Replace Array Subset(array=w628, new element=w621, index=w627) -> (w625:cluster{"time stamp":timestamp, "Y":dbl}[])
        n224 = Increment(x=w627) -> (x+1=w626:i32)
      }
    }
    "CO Sensitivity" <- w441
    n225 = case shown="True" w436 {
      tunnel: w435 -> [w608 w617]
      tunnel: w434 -> [w609 w616]
      tunnel: [w609 w615] -> w432
      tunnel: w428 -> [_ w614]
      tunnel: w431 -> [_ w613]
      tunnel: [w608 w612] -> w433
      tunnel: [w607 w611] -> w430
      tunnel: w431 -> [_ w611]
      tunnel: w429 -> [w607 _]
      frame False {
      }
      frame True {
        n226 = Bundle(w614, w613) -> (w610:cluster{timestamp, dbl})  [unwired: 1 in]
        n227 = Replace Array Subset(array=w617, new element=w610, index=w616) -> (w612:cluster{"time stamp":timestamp, "Y":dbl}[])
        n228 = Increment(x=w616) -> (x+1=w615:i32)
      }
    }
    "CO Zero" <- w433
    n229 = case shown="False" w427 {
      tunnel: w426 -> [_ w606]
      tunnel: [FALSE w603] -> w425
      frame False {
      }
      frame True {
        n230 = Select(t=FALSE, s=w606, f=TRUE) -> (s? t:f=w603:bool)
      }
    }
    "Network to cRIO live status" <- w425
    n231 = Wait (ms)(milliseconds to wait=u32 1000) -> ()  [unwired: 1 out]
  }
  n232 = Obtain Queue(name (unnamed)="FGGA_Command", element data type=w55) -> (queue out=w2:refnum<queue>, error out=w1:errorcluster)  [unwired: 3 in, 1 out]
  n233 = while {
    shift-right: [w632] -> _
    shift-left: u8 1 -> [w633]
    tunnel: w2 -> [w630]
    tunnel: w1 -> [w629]
    stop <- FALSE stop-if-true
    # "FGGA pump synchronise to WoW Wait on Wheel Flag"
    n234 = Wait (ms)(milliseconds to wait=u32 1000) -> ()  [unwired: 1 out]
    n235 = case shown="True" "FGGA pump\nsync to WoW" {
      tunnel: [w636 w641] -> w632
      tunnel: w633 -> [w636 w640]
      tunnel: w630 -> [_ w639]
      tunnel: w629 -> [_ w638]
      frame False {
      }
      frame True {
        n236 = local read "WoW Flag"() -> (w637:string)
        n237 = Scan Value(string=w637, format string="%d", default (0 dbl)=u8 0) -> (value=w641:u8)  [unwired: 1 out]
        n238 = Not Equal?(x=w641, y=w640) -> (x != y?=w644:bool)
        n239 = case shown="True" w644 {
          tunnel: w641 -> [_ w647]
          tunnel: w639 -> [_ w646]
          tunnel: w638 -> [_ w645]
          frame False {
          }
          frame True {
            n240 = Equal?(x=w647, y=u8 0) -> (x = y?=w652:bool)
            n241 = case shown="True" w652 {
              selector: w652 -> [w654 w655]
              tunnel: [w654 w655] -> w648
              frame False {
              }
              frame True {
              }
            }
            n242 = local write "FGGA Pump"(w648) -> ()
            n243 = Bundle(cluster=T4 {"Message"="", "Message Data"=variant} ("Message Cluster"), "Message"="FGGA_pump", "Message Data"=w648) -> (w649:T4)
            n244 = Enqueue Element(queue=w646, element=w649, error in (no error)=w645) -> ()  [unwired: 1 in, 3 out]
          }
        }
      }
    }
  }
  n245 = while {
    tunnel: w2 -> [w657]
    tunnel: w1 -> [w656]
    tunnel: [w659] -> _
    tunnel: w13 -> [w658]
    stop <- FALSE stop-if-true
    # "FGGA UI Event Handler Loop"
    n246 = event shown="[12] \"Flush Target Tank\": Value Change" {
      selector: _ -> [_ _ _ _ _ _ _ _ _ _ _ _ _ _ _ _ _]
      dyn-events: _ -> [_ _ _ _ _ _ _ _ _ _ _ _ _ _ _ _ _]
      timeout: _ -> [_ _ _ _ _ _ _ _ _ _ _ _ _ _ _ _ _]
      tunnel: w657 -> [w667 w671 w678 w685 w692 w699 w706 w713 w732 w841 w1014 w1081 w1148 w1205 w1292 w1360 w1367]
      tunnel: w656 -> [w666 w670 w677 w684 w691 w698 w705 w712 w731 w840 w1013 w1080 w1147 w1204 w1291 w1359 w1366]
      tunnel: [w661 w669 w676 w683 w690 w697 w704 w711 w718 w804 w1006 w1073 w1140 w1191 w1278 w1358 w1365] -> w659
      tunnel: w658 -> [_ _ _ _ _ _ _ _ _ w828 _ _ _ _ _ _ _]
      event "eV1": Value Change {
        n247 = event-data() -> ("NewVal"=w664:bool)  [unwired: 1 in]
        n248 = Bundle(cluster=T4 {"Message"="", "Message Data"=variant} ("Message Cluster"), "Message"="V1", "Message Data"=w664) -> (w662:T4)
        n249 = Enqueue Element(queue=w667, element=w662, error in (no error)=w666) -> (error out=w661:errorcluster)  [unwired: 1 in, 2 out]
      }
      event "eV2": Value Change {
        n250 = event-data() -> ("NewVal"=w668:bool)  [unwired: 1 in]
        n251 = Bundle(cluster=T4 {"Message"="", "Message Data"=variant} ("Message Cluster"), "Message"="V2", "Message Data"=w668) -> (w672:T4)
        n252 = Enqueue Element(queue=w671, element=w672, error in (no error)=w670) -> (error out=w669:errorcluster)  [unwired: 1 in, 2 out]
      }
      event "eV3": Value Change {
        n253 = event-data() -> ("NewVal"=w675:bool)  [unwired: 1 in]
        n254 = Bundle(cluster=T4 {"Message"="", "Message Data"=variant} ("Message Cluster"), "Message"="V3", "Message Data"=w675) -> (w679:T4)
        n255 = Enqueue Element(queue=w678, element=w679, error in (no error)=w677) -> (error out=w676:errorcluster)  [unwired: 1 in, 2 out]
      }
      event "eV4": Value Change {
        n256 = event-data() -> ("NewVal"=w682:bool)  [unwired: 1 in]
        n257 = Bundle(cluster=T4 {"Message"="", "Message Data"=variant} ("Message Cluster"), "Message"="V4", "Message Data"=w682) -> (w686:T4)
        n258 = Enqueue Element(queue=w685, element=w686, error in (no error)=w684) -> (error out=w683:errorcluster)  [unwired: 1 in, 2 out]
      }
      event "FGGA Pump": Value Change {
        n259 = event-data() -> ("NewVal"=w689:bool)  [unwired: 1 in]
        n260 = Bundle(cluster=T4 {"Message"="", "Message Data"=variant} ("Message Cluster"), "Message"="FGGA_pump", "Message Data"=w689) -> (w693:T4)
        n261 = Enqueue Element(queue=w692, element=w693, error in (no error)=w691) -> (error out=w690:errorcluster)  [unwired: 1 in, 2 out]
      }
      event "Confirm Flight Number": Value Change {
        n262 = event-data() -> ()  [unwired: 1 in, 6 out]
        n263 = local read "Flight Number"() -> (w696:string)
        n264 = Bundle(cluster=T4 {"Message"="", "Message Data"=variant} ("Message Cluster"), "Message"="Flight Number", "Message Data"=w696) -> (w700:T4)
        n265 = Enqueue Element(queue=w699, element=w700, error in (no error)=w698) -> (error out=w697:errorcluster)  [unwired: 1 in, 2 out]
      }
      event "FGGA Restart": Value Change {
        n266 = event-data() -> ("NewVal"=w703:bool)  [unwired: 1 in]
        n267 = Bundle(cluster=T4 {"Message"="", "Message Data"=variant} ("Message Cluster"), "Message"="FGGA_restart", "Message Data"=w703) -> (w707:T4)
        n268 = Enqueue Element(queue=w706, element=w707, error in (no error)=w705) -> (error out=w704:errorcluster)  [unwired: 1 in, 2 out]
      }
      event "cRIO File IO Stop\n(USB Flash Drive Unmount)": Value Change {
        n269 = event-data() -> ("NewVal"=w710:bool)  [unwired: 1 in]
        n270 = Bundle(cluster=T4 {"Message"="", "Message Data"=variant} ("Message Cluster"), "Message"="Stop File Write", "Message Data"=w710) -> (w714:T4)
        n271 = Enqueue Element(queue=w713, element=w714, error in (no error)=w712) -> (error out=w711:errorcluster)  [unwired: 1 in, 2 out]
      }
      event "High Cal": Value Change {
        n272 = event-data() -> ()  [unwired: 1 in, 1 out]
        n273 = flat-sequence {
          tunnel: w732 -> [w737]
          tunnel: w731 -> [w736]
          tunnel: [w735] -> w730
          tunnel: [w734] -> w729
          tunnel: w730 -> [w753]
          tunnel: w729 -> [w752]
          tunnel: [w750] -> w727
          tunnel: [w749] -> w725
          tunnel: [w758] -> w728
          tunnel: w727 -> [w758]
          tunnel: [w757] -> w726
          tunnel: w725 -> [w757]
          tunnel: w728 -> [w768]
          tunnel: w726 -> [w767]
          tunnel: [w765] -> w723
          tunnel: [w764] -> w721
          tunnel: [w774] -> w724
          tunnel: w723 -> [w774]
          tunnel: [w773] -> w722
          tunnel: w721 -> [w773]
          tunnel: w724 -> [w784]
          tunnel: w722 -> [w783]
          tunnel: [w781] -> w720
          tunnel: [w780] -> w719
          tunnel: w720 -> [w798]
          tunnel: w719 -> [w797]
          tunnel: [w795] -> w717
          tunnel: [w803] -> w718
          tunnel: w717 -> [w803]
          frame #0 {
            w733 = TRUE
            n274 = Cluster To Array(cluster=T11 {"Message"="V2", "Message 2"="V3", "Message 3"="V4"}) -> (array=w738:string[])
            n275 = for {
              tunnel: w738 -> [w745] mode=indexing
              tunnel: w737 -> [w744]
              tunnel: w736 -> [w743]
              tunnel: [w742] -> w735
              tunnel: [w741] -> w734
              tunnel: w733 -> [w740]
              n276 = Bundle(cluster=T4 {"Message"="", "Message Data"=variant} ("Message Cluster"), "Message"=w745, "Message Data"=w740) -> (w747:T4)
              n277 = Enqueue Element(queue=w744, element=w747, error in (no error)=w743) -> (queue out=w742:refnum<queue>, error out=w741:errorcluster)  [unwired: 1 in, 1 out]
            }
            n278 = local write "eV2"(w733) -> ()
            n279 = local write "eV4"(w733) -> ()
            n280 = local write "eV3"(w733) -> ()
          }
          frame #1 {
            n281 = local read "MFC_1 User Set Value"() -> (w748:dbl)
            n282 = local write "MFC_1\nSLPM Value"(w748) -> ()
            n283 = Bundle(cluster=T4 {"Message"="", "Message Data"=variant} ("Message Cluster"), "Message"="MFC_1", "Message Data"=w748) -> (w751:T4)
            n284 = Enqueue Element(queue=w753, element=w751, error in (no error)=w752) -> (queue out=w750:refnum<queue>, error out=w749:errorcluster)  [unwired: 1 in, 1 out]
          }
          frame #2 {
            n285 = for {
              N: 45 -> [w762]
              i -> [w761]
              n286 = Subtract(x=w762, y=w761) -> (x-y=w760:i32)
              n287 = Decrement(x=w760) -> (x-1=→"High Cal\nFlush Time Remain (sec)":i32)
              n288 = Wait (ms)(milliseconds to wait=u32 1000) -> ()  [unwired: 1 out]
            }
          }
          frame #3 {
            w766 = TRUE
            n289 = Bundle(cluster=T4 {"Message"="", "Message Data"=variant} ("Message Cluster"), "Message"="V1", "Message Data"=w766) -> (w769:T4)
            n290 = local write "eV1"(w766) -> ()
            n291 = Enqueue Element(queue=w768, element=w769, error in (no error)=w767) -> (queue out=w765:refnum<queue>, error out=w764:errorcluster)  [unwired: 1 in, 1 out]
          }
          frame #4 {
            n292 = for {
              N: 60 -> [w778]
              i -> [w777]
              n293 = Subtract(x=w778, y=w777) -> (x-y=w776:i32)
              n294 = Decrement(x=w776) -> (x-1=→"High Cal\nCal Time Remain (sec)":i32)
              n295 = Wait (ms)(milliseconds to wait=u32 1000) -> ()  [unwired: 1 out]
            }
          }
          frame #5 {
            w782 = FALSE
            n296 = Cluster To Array(cluster=T12 {"Message"="V2", "Message 2"="V3", "Message 3"="V4", "Message 4"="V1"}) -> (array=w785:string[])
            n297 = for {
              tunnel: w785 -> [w792] mode=indexing
              tunnel: [w791] -> w781
              tunnel: [w790] -> w780
              tunnel: w782 -> [w789]
              tunnel: w784 -> [w788]
              tunnel: w783 -> [w787]
              n298 = Bundle(cluster=T4 {"Message"="", "Message Data"=variant} ("Message Cluster"), "Message"=w792, "Message Data"=w789) -> (w794:T4)
              n299 = Enqueue Element(queue=w788, element=w794, error in (no error)=w787) -> (queue out=w791:refnum<queue>, error out=w790:errorcluster)  [unwired: 1 in, 1 out]
            }
            n300 = local write "eV2"(w782) -> ()
            n301 = local write "eV4"(w782) -> ()
            n302 = local write "eV3"(w782) -> ()
            n303 = local write "eV1"(w782) -> ()
          }
          frame #6 {
            w796 = 0.0 ("MFC_1\nSLPM Value")
            n304 = local write "MFC_1\nSLPM Value"(w796) -> ()
            n305 = Bundle(cluster=T4 {"Message"="", "Message Data"=variant} ("Message Cluster"), "Message"="MFC_1", "Message Data"=w796) -> (w800:T4)
            n306 = Enqueue Element(queue=w798, element=w800, error in (no error)=w797) -> (error out=w795:errorcluster)  [unwired: 1 in, 2 out]
          }
          frame #7 {
            n307 = local write "High Cal"(FALSE ("High Cal")) -> ()
          }
        }
      }
      event "Span Cal": Value Change {
        n308 = event-data() -> ()  [unwired: 1 in, 1 out]
        n309 = flat-sequence {
          tunnel: w841 -> [w847]
          tunnel: w840 -> [w846]
          tunnel: [w845] -> w839
          tunnel: [w844] -> w838
          tunnel: w839 -> [w863]
          tunnel: w838 -> [w862]
          tunnel: [w860] -> w836
          tunnel: [w859] -> w834
          tunnel: [w868] -> w837
          tunnel: w836 -> [w868]
          tunnel: [w867] -> w835
          tunnel: w834 -> [w867]
          tunnel: w837 -> [w874]
          tunnel: w835 -> [w875]
          tunnel: [w875] -> w810
          tunnel: w828 -> [w876]
          tunnel: [w876] -> w808
          tunnel: [w874] -> w806
          tunnel: w810 -> [w884]
          tunnel: [w884] -> w809
          tunnel: w808 -> [w883]
          tunnel: [w883] -> w807
          tunnel: w806 -> [w881]
          tunnel: [w881] -> w805
          tunnel: [w885] -> w827
          tunnel: w809 -> [w888]
          tunnel: [w887] -> w826
          tunnel: w807 -> [w897]
          tunnel: w805 -> [w886]
          tunnel: [w900] -> w833
          tunnel: w827 -> [w900]
          tunnel: [w899] -> w832
          tunnel: w826 -> [w899]
          tunnel: w833 -> [w910]
          tunnel: w832 -> [w909]
          tunnel: [w907] -> w831
          tunnel: [w906] -> w830
          tunnel: w831 -> [w925]
          tunnel: w830 -> [w924]
          tunnel: [w922] -> w829
          tunnel: [w921] -> w823
          tunnel: w829 -> [w931]
          tunnel: [w931] -> w825
          tunnel: [w929] -> w824
          tunnel: w823 -> [w929]
          tunnel: w825 -> [w936]
          tunnel: w824 -> [w938]
          tunnel: [w935] -> w822
          tunnel: [w932] -> w821
          tunnel: w822 -> [w952]
          tunnel: w821 -> [w950]
          tunnel: [w949] -> w820
          tunnel: [w948] -> w817
          tunnel: w820 -> [w957]
          tunnel: [w957] -> w819
          tunnel: [w956] -> w818
          tunnel: w817 -> [w956]
          tunnel: w819 -> [w969]
          tunnel: w818 -> [w967]
          tunnel: [w965] -> w815
          tunnel: [w964] -> w813
          tunnel: [w973] -> w816
          tunnel: w815 -> [w973]
          tunnel: [w972] -> w814
          tunnel: w813 -> [w972]
          tunnel: w816 -> [w984]
          tunnel: w814 -> [w983]
          tunnel: [w981] -> w812
          tunnel: [w980] -> w811
          tunnel: w812 -> [w999]
          tunnel: w811 -> [w998]
          tunnel: [w995] -> w804
          frame #0 {
            w843 = TRUE
            n310 = Cluster To Array(cluster=T11 {"Message"="V2", "Message 2"="V3", "Message 3"="V4"}) -> (array=w848:string[])
            n311 = for {
              tunnel: w848 -> [w855] mode=indexing
              tunnel: w847 -> [w854]
              tunnel: w846 -> [w853]
              tunnel: [w852] -> w845
              tunnel: [w851] -> w844
              tunnel: w843 -> [w850]
              n312 = Bundle(cluster=T4 {"Message"="", "Message Data"=variant} ("Message Cluster"), "Message"=w855, "Message Data"=w850) -> (w857:T4)
              n313 = Enqueue Element(queue=w854, element=w857, error in (no error)=w853) -> (queue out=w852:refnum<queue>, error out=w851:errorcluster)  [unwired: 1 in, 1 out]
            }
            n314 = local write "High Cal"(TRUE ("High Cal")) -> ()
            n315 = local write "eV2"(w843) -> ()
            n316 = local write "eV4"(w843) -> ()
            n317 = local write "eV3"(w843) -> ()
          }
          frame #1 {
            n318 = local read "MFC_1 User Set Value"() -> (w858:dbl)
            n319 = local write "MFC_1\nSLPM Value"(w858) -> ()
            n320 = Bundle(cluster=T4 {"Message"="", "Message Data"=variant} ("Message Cluster"), "Message"="MFC_1", "Message Data"=w858) -> (w861:T4)
            n321 = Enqueue Element(queue=w863, element=w861, error in (no error)=w862) -> (queue out=w860:refnum<queue>, error out=w859:errorcluster)  [unwired: 1 in, 1 out]
          }
          frame #2 {
            n322 = for {
              N: 45 -> [w872]
              i -> [w871]
              n323 = Subtract(x=w872, y=w871) -> (x-y=w870:i32)
              n324 = Decrement(x=w870) -> (x-1=w869:i32)
              n325 = local write "High Cal\nFlush Time Remain (sec)"(w869) -> ()
              n326 = Wait (ms)(milliseconds to wait=u32 1000) -> ()  [unwired: 1 out]
            }
          }
          frame #3 {
            n327 = Bundle(cluster=T4 {"Message"="", "Message Data"=variant} ("Message Cluster"), "Message"="CO CAL", "Message Data"=TRUE) -> (w878:T4)
            n328 = Enqueue Element(queue=w876, element=w878) -> ()  [unwired: 2 in, 3 out]
          }
          frame #4 {
            # "To Ensure\nCO CAL\nis certain"
            n329 = Wait (ms)(milliseconds to wait=u32 1000) -> ()  [unwired: 1 out]
          }
          frame #5 {
            w892 = TRUE
            n330 = Bundle(cluster=T4 {"Message"="", "Message Data"=variant} ("Message Cluster"), "Message"="CO CAL", "Message Data"=FALSE) -> (w893:T4)
            n331 = Bundle(cluster=T4 {"Message"="", "Message Data"=variant} ("Message Cluster"), "Message"="V1", "Message Data"=w892) -> (w891:T4)
            n332 = local write "eV1"(w892) -> ()
            n333 = Enqueue Element(queue=w897, element=w893) -> ()  [unwired: 2 in, 3 out]
            n334 = Enqueue Element(queue=w886, element=w891, error in (no error)=w888) -> (queue out=w885:refnum<queue>, error out=w887:errorcluster)  [unwired: 1 in, 1 out]
          }
          frame #6 {
            n335 = for {
              N: 60 -> [w904]
              i -> [w903]
              n336 = Subtract(x=w904, y=w903) -> (x-y=w902:i32)
              n337 = Decrement(x=w902) -> (x-1=w901:i32)
              n338 = local write "High Cal\nCal Time Remain (sec)"(w901) -> ()
              n339 = Wait (ms)(milliseconds to wait=u32 1000) -> ()  [unwired: 1 out]
            }
          }
          frame #7 {
            w908 = FALSE
            n340 = Cluster To Array(cluster=T12 {"Message"="V2", "Message 2"="V3", "Message 3"="V4", "Message 4"="V1"}) -> (array=w911:string[])
            n341 = for {
              tunnel: w911 -> [w918] mode=indexing
              tunnel: [w917] -> w907
              tunnel: [w916] -> w906
              tunnel: w908 -> [w915]
              tunnel: w910 -> [w914]
              tunnel: w909 -> [w913]
              n342 = Bundle(cluster=T4 {"Message"="", "Message Data"=variant} ("Message Cluster"), "Message"=w918, "Message Data"=w915) -> (w920:T4)
              n343 = Enqueue Element(queue=w914, element=w920, error in (no error)=w913) -> (queue out=w917:refnum<queue>, error out=w916:errorcluster)  [unwired: 1 in, 1 out]
            }
            n344 = local write "eV2"(w908) -> ()
            n345 = local write "eV4"(w908) -> ()
            n346 = local write "eV3"(w908) -> ()
            n347 = local write "eV1"(w908) -> ()
          }
          frame #8 {
            w923 = 0.0 ("MFC_1\nSLPM Value")
            n348 = local write "MFC_1\nSLPM Value"(w923) -> ()
            n349 = Bundle(cluster=T4 {"Message"="", "Message Data"=variant} ("Message Cluster"), "Message"="MFC_1", "Message Data"=w923) -> (w927:T4)
            n350 = Enqueue Element(queue=w925, element=w927, error in (no error)=w924) -> (queue out=w921:refnum<queue>, error out=w922:errorcluster)  [unwired: 1 in, 1 out]
          }
          frame #9 {
            n351 = local write "High Cal"(FALSE ("High Cal")) -> ()
          }
          frame #10 {
            w933 = TRUE
            n352 = Cluster To Array(cluster=cluster{"Message":string, "Message 3":string} {"Message"="V2", "Message 3"="V4"}) -> (array=w939:string[])
            n353 = for {
              tunnel: w939 -> [w945] mode=indexing
              tunnel: w938 -> [w944]
              tunnel: [w943] -> w932
              tunnel: [w942] -> w935
              tunnel: w933 -> [w941]
              tunnel: w936 -> [w940]
              n354 = Bundle(cluster=T4 {"Message"="", "Message Data"=variant} ("Message Cluster"), "Message"=w945, "Message Data"=w941) -> (w947:T4)
              n355 = Enqueue Element(queue=w944, element=w947, error in (no error)=w940) -> (queue out=w943:refnum<queue>, error out=w942:errorcluster)  [unwired: 1 in, 1 out]
            }
            n356 = local write "eV4"(w933) -> ()
            n357 = local write "eV2"(w933) -> ()
            n358 = local write "Low Cal"(TRUE ("Low Cal")) -> ()
          }
          frame #11 {
            n359 = local read "MFC_1 User Set Value"() -> (w953:dbl)
            n360 = local write "MFC_1\nSLPM Value"(w953) -> ()
            n361 = Bundle(cluster=T4 {"Message"="", "Message Data"=variant} ("Message Cluster"), "Message"="MFC_1", "Message Data"=w953) -> (w954:T4)
            n362 = Enqueue Element(queue=w950, element=w954, error in (no error)=w952) -> (queue out=w949:refnum<queue>, error out=w948:errorcluster)  [unwired: 1 in, 1 out]
          }
          frame #12 {
            n363 = for {
              N: 45 -> [w962]
              i -> [w961]
              n364 = Subtract(x=w962, y=w961) -> (x-y=w960:i32)
              n365 = Decrement(x=w960) -> (x-1=w959:i32)
              n366 = local write "Low Cal\nFlush Time Remain (sec)"(w959) -> ()
              n367 = Wait (ms)(milliseconds to wait=u32 1000) -> ()  [unwired: 1 out]
            }
          }
          frame #13 {
            w966 = TRUE
            n368 = local write "eV1"(w966) -> ()
            n369 = Bundle(cluster=T4 {"Message"="", "Message Data"=variant} ("Message Cluster"), "Message"="V1", "Message Data"=w966) -> (w970:T4)
            n370 = Enqueue Element(queue=w969, element=w970, error in (no error)=w967) -> (queue out=w965:refnum<queue>, error out=w964:errorcluster)  [unwired: 1 in, 1 out]
          }
          frame #14 {
            n371 = for {
              N: 60 -> [w978]
              i -> [w977]
              n372 = Subtract(x=w978, y=w977) -> (x-y=w976:i32)
              n373 = Decrement(x=w976) -> (x-1=w975:i32)
              n374 = local write "Low Cal\nCal Time Remain (sec)"(w975) -> ()
              n375 = Wait (ms)(milliseconds to wait=u32 1000) -> ()  [unwired: 1 out]
            }
          }
          frame #15 {
            w982 = FALSE
            n376 = Cluster To Array(cluster=T13 {"Message"="V2", "Message 3"="V4", "Message 4"="V1"}) -> (array=w985:string[])
            n377 = local write "eV1"(w982) -> ()
            n378 = local write "eV2"(w982) -> ()
            n379 = local write "eV4"(w982) -> ()
            n380 = for {
              tunnel: w985 -> [w992] mode=indexing
              tunnel: [w991] -> w981
              tunnel: [w990] -> w980
              tunnel: w982 -> [w989]
              tunnel: w984 -> [w988]
              tunnel: w983 -> [w987]
              n381 = Bundle(cluster=T4 {"Message"="", "Message Data"=variant} ("Message Cluster"), "Message"=w992, "Message Data"=w989) -> (w994:T4)
              n382 = Enqueue Element(queue=w988, element=w994, error in (no error)=w987) -> (queue out=w991:refnum<queue>, error out=w990:errorcluster)  [unwired: 1 in, 1 out]
            }
          }
          frame #16 {
            w996 = FALSE
            w997 = 0.0 ("MFC_1\nSLPM Value")
            n383 = local write "MFC_1\nSLPM Value"(w997) -> ()
            n384 = local write "Span Cal"(w996) -> ()
            n385 = local write "Low Cal"(w996) -> ()
            n386 = Bundle(cluster=T4 {"Message"="", "Message Data"=variant} ("Message Cluster"), "Message"="MFC_1", "Message Data"=w997) -> (w1001:T4)
            n387 = Enqueue Element(queue=w999, element=w1001, error in (no error)=w998) -> (error out=w995:errorcluster)  [unwired: 1 in, 2 out]
          }
        }
      }
      event "Flush High Tank": Value Change {
        n388 = event-data() -> ()  [unwired: 1 in, 1 out]
        n389 = flat-sequence {
          tunnel: w1014 -> [w1019]
          tunnel: w1013 -> [w1018]
          tunnel: [w1017] -> w1012
          tunnel: [w1016] -> w1011
          tunnel: w1012 -> [w1035]
          tunnel: w1011 -> [w1034]
          tunnel: [w1032] -> w1010
          tunnel: [w1031] -> w1009
          tunnel: w1010 -> [w1038]
          tunnel: w1009 -> [w1039]
          tunnel: [w1039] -> w1004
          tunnel: [w1038] -> w1003
          tunnel: [w1049] -> w1008
          tunnel: [w1048] -> w1007
          tunnel: w1004 -> [w1047]
          tunnel: w1003 -> [w1046]
          tunnel: w1008 -> [w1064]
          tunnel: w1007 -> [w1063]
          tunnel: [w1061] -> w1005
          tunnel: [w1069] -> w1006
          tunnel: w1005 -> [w1069]
          frame #0 {
            w1015 = TRUE
            n390 = Cluster To Array(cluster=T11 {"Message"="V2", "Message 2"="V3", "Message 3"="V4"}) -> (array=w1020:string[])
            n391 = for {
              tunnel: w1020 -> [w1027] mode=indexing
              tunnel: w1019 -> [w1026]
              tunnel: w1018 -> [w1025]
              tunnel: [w1024] -> w1017
              tunnel: [w1023] -> w1016
              tunnel: w1015 -> [w1022]
              n392 = Bundle(cluster=T4 {"Message"="", "Message Data"=variant} ("Message Cluster"), "Message"=w1027, "Message Data"=w1022) -> (w1029:T4)
              n393 = Enqueue Element(queue=w1026, element=w1029, error in (no error)=w1025) -> (queue out=w1024:refnum<queue>, error out=w1023:errorcluster)  [unwired: 1 in, 1 out]
            }
            n394 = local write "eV2"(w1015) -> ()
            n395 = local write "eV4"(w1015) -> ()
            n396 = local write "eV3"(w1015) -> ()
          }
          frame #1 {
            n397 = local read "MFC_1 User Set Value"() -> (w1030:dbl)
            n398 = local write "MFC_1\nSLPM Value"(w1030) -> ()
            n399 = Bundle(cluster=T4 {"Message"="", "Message Data"=variant} ("Message Cluster"), "Message"="MFC_1", "Message Data"=w1030) -> (w1033:T4)
            n400 = Enqueue Element(queue=w1035, element=w1033, error in (no error)=w1034) -> (queue out=w1032:refnum<queue>, error out=w1031:errorcluster)  [unwired: 1 in, 1 out]
          }
          frame #2 {
            n401 = for {
              N: 15 -> [w1044]
              i -> [w1043]
              n402 = Subtract(x=w1044, y=w1043) -> (x-y=w1042:i32)
              n403 = Decrement(x=w1042) -> (x-1=→"Flush High Tank\nTime Remain (sec)":i32)
              n404 = Wait (ms)(milliseconds to wait=u32 1000) -> ()  [unwired: 1 out]
            }
          }
          frame #3 {
            w1050 = FALSE
            n405 = Cluster To Array(cluster=T11 {"Message"="V2", "Message 2"="V3", "Message 3"="V4"}) -> (array=w1051:string[])
            n406 = for {
              tunnel: w1051 -> [w1058] mode=indexing
              tunnel: [w1057] -> w1049
              tunnel: [w1056] -> w1048
              tunnel: w1050 -> [w1055]
              tunnel: w1046 -> [w1054]
              tunnel: w1047 -> [w1053]
              n407 = Bundle(cluster=T4 {"Message"="", "Message Data"=variant} ("Message Cluster"), "Message"=w1058, "Message Data"=w1055) -> (w1060:T4)
              n408 = Enqueue Element(queue=w1054, element=w1060, error in (no error)=w1053) -> (queue out=w1057:refnum<queue>, error out=w1056:errorcluster)  [unwired: 1 in, 1 out]
            }
            n409 = local write "eV2"(w1050) -> ()
            n410 = local write "eV4"(w1050) -> ()
            n411 = local write "eV3"(w1050) -> ()
          }
          frame #4 {
            w1062 = 0.0 ("MFC_1\nSLPM Value")
            n412 = local write "MFC_1\nSLPM Value"(w1062) -> ()
            n413 = Bundle(cluster=T4 {"Message"="", "Message Data"=variant} ("Message Cluster"), "Message"="MFC_1", "Message Data"=w1062) -> (w1066:T4)
            n414 = Enqueue Element(queue=w1064, element=w1066, error in (no error)=w1063) -> (error out=w1061:errorcluster)  [unwired: 1 in, 2 out]
          }
          frame #5 {
            n415 = local write "Flush High Tank"(FALSE ("High Cal")) -> ()
          }
        }
      }
      event "Flush Low Tank": Value Change {
        n416 = event-data() -> ()  [unwired: 1 in, 1 out]
        n417 = flat-sequence {
          tunnel: w1081 -> [w1086]
          tunnel: w1080 -> [w1085]
          tunnel: [w1084] -> w1079
          tunnel: [w1083] -> w1078
          tunnel: w1079 -> [w1102]
          tunnel: w1078 -> [w1101]
          tunnel: [w1099] -> w1077
          tunnel: [w1098] -> w1076
          tunnel: w1077 -> [w1105]
          tunnel: w1076 -> [w1106]
          tunnel: [w1106] -> w1071
          tunnel: [w1105] -> w1070
          tunnel: [w1116] -> w1075
          tunnel: [w1115] -> w1074
          tunnel: w1071 -> [w1114]
          tunnel: w1070 -> [w1113]
          tunnel: w1075 -> [w1131]
          tunnel: w1074 -> [w1130]
          tunnel: [w1128] -> w1072
          tunnel: [w1136] -> w1073
          tunnel: w1072 -> [w1136]
          frame #0 {
            w1082 = TRUE
            n418 = Cluster To Array(cluster=cluster{"Message":string, "Message 3":string} {"Message"="V2", "Message 3"="V4"}) -> (array=w1087:string[])
            n419 = for {
              tunnel: w1087 -> [w1094] mode=indexing
              tunnel: w1086 -> [w1093]
              tunnel: w1085 -> [w1092]
              tunnel: [w1091] -> w1084
              tunnel: [w1090] -> w1083
              tunnel: w1082 -> [w1089]
              n420 = Bundle(cluster=T4 {"Message"="", "Message Data"=variant} ("Message Cluster"), "Message"=w1094, "Message Data"=w1089) -> (w1096:T4)
              n421 = Enqueue Element(queue=w1093, element=w1096, error in (no error)=w1092) -> (queue out=w1091:refnum<queue>, error out=w1090:errorcluster)  [unwired: 1 in, 1 out]
            }
            n422 = local write "eV2"(w1082) -> ()
            n423 = local write "eV4"(w1082) -> ()
          }
          frame #1 {
            n424 = local read "MFC_1 User Set Value"() -> (w1097:dbl)
            n425 = local write "MFC_1\nSLPM Value"(w1097) -> ()
            n426 = Bundle(cluster=T4 {"Message"="", "Message Data"=variant} ("Message Cluster"), "Message"="MFC_1", "Message Data"=w1097) -> (w1100:T4)
            n427 = Enqueue Element(queue=w1102, element=w1100, error in (no error)=w1101) -> (queue out=w1099:refnum<queue>, error out=w1098:errorcluster)  [unwired: 1 in, 1 out]
          }
          frame #2 {
            n428 = for {
              N: 15 -> [w1111]
              i -> [w1110]
              n429 = Subtract(x=w1111, y=w1110) -> (x-y=w1109:i32)
              n430 = Decrement(x=w1109) -> (x-1=→"Flush Low Tank\nTime Remain (sec)":i32)
              n431 = Wait (ms)(milliseconds to wait=u32 1000) -> ()  [unwired: 1 out]
            }
          }
          frame #3 {
            w1117 = FALSE
            n432 = Cluster To Array(cluster=cluster{"Message":string, "Message 3":string} {"Message"="V2", "Message 3"="V4"}) -> (array=w1118:string[])
            n433 = for {
              tunnel: w1118 -> [w1125] mode=indexing
              tunnel: [w1124] -> w1116
              tunnel: [w1123] -> w1115
              tunnel: w1117 -> [w1122]
              tunnel: w1113 -> [w1121]
              tunnel: w1114 -> [w1120]
              n434 = Bundle(cluster=T4 {"Message"="", "Message Data"=variant} ("Message Cluster"), "Message"=w1125, "Message Data"=w1122) -> (w1127:T4)
              n435 = Enqueue Element(queue=w1121, element=w1127, error in (no error)=w1120) -> (queue out=w1124:refnum<queue>, error out=w1123:errorcluster)  [unwired: 1 in, 1 out]
            }
            n436 = local write "eV2"(w1117) -> ()
            n437 = local write "eV4"(w1117) -> ()
          }
          frame #4 {
            w1129 = 0.0 ("MFC_1\nSLPM Value")
            n438 = local write "MFC_1\nSLPM Value"(w1129) -> ()
            n439 = Bundle(cluster=T4 {"Message"="", "Message Data"=variant} ("Message Cluster"), "Message"="MFC_1", "Message Data"=w1129) -> (w1133:T4)
            n440 = Enqueue Element(queue=w1131, element=w1133, error in (no error)=w1130) -> (error out=w1128:errorcluster)  [unwired: 1 in, 2 out]
          }
          frame #5 {
            n441 = local write "Flush Low Tank"(FALSE ("High Cal")) -> ()
          }
        }
      }
      event "Flush Target Tank": Value Change {
        n442 = event-data() -> ()  [unwired: 1 in, 1 out]
        n443 = flat-sequence {
          tunnel: w1148 -> [w1156]
          tunnel: w1147 -> [w1155]
          tunnel: [w1154] -> w1146
          tunnel: [w1153] -> w1145
          tunnel: w1146 -> [w1162]
          tunnel: w1145 -> [w1161]
          tunnel: [w1159] -> w1144
          tunnel: [w1158] -> w1143
          tunnel: w1144 -> [w1165]
          tunnel: w1143 -> [w1166]
          tunnel: [w1166] -> w1138
          tunnel: [w1165] -> w1137
          tunnel: [w1179] -> w1142
          tunnel: [w1178] -> w1141
          tunnel: w1138 -> [w1177]
          tunnel: w1137 -> [w1176]
          tunnel: w1142 -> [w1184]
          tunnel: w1141 -> [w1183]
          tunnel: [w1181] -> w1139
          tunnel: [w1189] -> w1140
          tunnel: w1139 -> [w1189]
          frame #0 {
            w1152 = TRUE
            n444 = local write "eV4"(w1152) -> ()
            n445 = Bundle(cluster=T4 {"Message"="", "Message Data"=variant} ("Message Cluster"), "Message"="V4" ("Message 3"), "Message Data"=w1152) -> (w1151:T4)
            n446 = Enqueue Element(queue=w1156, element=w1151, error in (no error)=w1155) -> (queue out=w1154:refnum<queue>, error out=w1153:errorcluster)  [unwired: 1 in, 1 out]
          }
          frame #1 {
            n447 = local read "MFC_1 User Set Value"() -> (w1157:dbl)
            n448 = local write "MFC_1\nSLPM Value"(w1157) -> ()
            n449 = Bundle(cluster=T4 {"Message"="", "Message Data"=variant} ("Message Cluster"), "Message"="MFC_1", "Message Data"=w1157) -> (w1160:T4)
            n450 = Enqueue Element(queue=w1162, element=w1160, error in (no error)=w1161) -> (queue out=w1159:refnum<queue>, error out=w1158:errorcluster)  [unwired: 1 in, 1 out]
          }
          frame #2 {
            n451 = for {
              N: 15 -> [w1171]
              i -> [w1170]
              n452 = Subtract(x=w1171, y=w1170) -> (x-y=w1169:i32)
              n453 = Decrement(x=w1169) -> (x-1=→"Flush Target Tank\nTime Remain (sec)":i32)
              n454 = Wait (ms)(milliseconds to wait=u32 1000) -> ()  [unwired: 1 out]
            }
          }
          frame #3 {
            w1180 = FALSE
            n455 = Bundle(cluster=T4 {"Message"="", "Message Data"=variant} ("Message Cluster"), "Message"="V4" ("Message 3"), "Message Data"=w1180) -> (w1175:T4)
            n456 = local write "eV4"(w1180) -> ()
            n457 = Enqueue Element(queue=w1176, element=w1175, error in (no error)=w1177) -> (queue out=w1179:refnum<queue>, error out=w1178:errorcluster)  [unwired: 1 in, 1 out]
          }
          frame #4 {
            w1182 = 0.0 ("MFC_1\nSLPM Value")
            n458 = local write "MFC_1\nSLPM Value"(w1182) -> ()
            n459 = Bundle(cluster=T4 {"Message"="", "Message Data"=variant} ("Message Cluster"), "Message"="MFC_1", "Message Data"=w1182) -> (w1186:T4)
            n460 = Enqueue Element(queue=w1184, element=w1186, error in (no error)=w1183) -> (error out=w1181:errorcluster)  [unwired: 1 in, 2 out]
          }
          frame #5 {
            n461 = local write "Flush Target Tank"(FALSE ("High Cal")) -> ()
          }
        }
      }
      event "Low Cal": Value Change {
        n462 = event-data() -> ()  [unwired: 1 in, 1 out]
        n463 = flat-sequence {
          tunnel: w1205 -> [w1210]
          tunnel: w1204 -> [w1209]
          tunnel: [w1208] -> w1203
          tunnel: [w1207] -> w1202
          tunnel: w1203 -> [w1226]
          tunnel: w1202 -> [w1225]
          tunnel: [w1223] -> w1200
          tunnel: [w1222] -> w1198
          tunnel: [w1231] -> w1201
          tunnel: w1200 -> [w1231]
          tunnel: [w1230] -> w1199
          tunnel: w1198 -> [w1230]
          tunnel: w1201 -> [w1241]
          tunnel: w1199 -> [w1240]
          tunnel: [w1238] -> w1196
          tunnel: [w1237] -> w1194
          tunnel: [w1247] -> w1197
          tunnel: w1196 -> [w1247]
          tunnel: [w1246] -> w1195
          tunnel: w1194 -> [w1246]
          tunnel: w1197 -> [w1257]
          tunnel: w1195 -> [w1256]
          tunnel: [w1254] -> w1193
          tunnel: [w1253] -> w1192
          tunnel: w1193 -> [w1271]
          tunnel: w1192 -> [w1270]
          tunnel: [w1268] -> w1190
          tunnel: [w1276] -> w1191
          tunnel: w1190 -> [w1276]
          frame #0 {
            w1206 = TRUE
            n464 = Cluster To Array(cluster=cluster{"Message":string, "Message 3":string} {"Message"="V2", "Message 3"="V4"}) -> (array=w1211:string[])
            n465 = for {
              tunnel: w1211 -> [w1218] mode=indexing
              tunnel: w1210 -> [w1217]
              tunnel: w1209 -> [w1216]
              tunnel: [w1215] -> w1208
              tunnel: [w1214] -> w1207
              tunnel: w1206 -> [w1213]
              n466 = Bundle(cluster=T4 {"Message"="", "Message Data"=variant} ("Message Cluster"), "Message"=w1218, "Message Data"=w1213) -> (w1220:T4)
              n467 = Enqueue Element(queue=w1217, element=w1220, error in (no error)=w1216) -> (queue out=w1215:refnum<queue>, error out=w1214:errorcluster)  [unwired: 1 in, 1 out]
            }
            n468 = local write "eV2"(w1206) -> ()
            n469 = local write "eV4"(w1206) -> ()
          }
          frame #1 {
            n470 = local read "MFC_1 User Set Value"() -> (w1221:dbl)
            n471 = local write "MFC_1\nSLPM Value"(w1221) -> ()
            n472 = Bundle(cluster=T4 {"Message"="", "Message Data"=variant} ("Message Cluster"), "Message"="MFC_1", "Message Data"=w1221) -> (w1224:T4)
            n473 = Enqueue Element(queue=w1226, element=w1224, error in (no error)=w1225) -> (queue out=w1223:refnum<queue>, error out=w1222:errorcluster)  [unwired: 1 in, 1 out]
          }
          frame #2 {
            n474 = for {
              N: 45 -> [w1235]
              i -> [w1234]
              n475 = Subtract(x=w1235, y=w1234) -> (x-y=w1233:i32)
              n476 = Decrement(x=w1233) -> (x-1=→"Low Cal\nFlush Time Remain (sec)":i32)
              n477 = Wait (ms)(milliseconds to wait=u32 1000) -> ()  [unwired: 1 out]
            }
          }
          frame #3 {
            w1239 = TRUE
            n478 = Bundle(cluster=T4 {"Message"="", "Message Data"=variant} ("Message Cluster"), "Message"="V1", "Message Data"=w1239) -> (w1242:T4)
            n479 = local write "eV1"(w1239) -> ()
            n480 = Enqueue Element(queue=w1241, element=w1242, error in (no error)=w1240) -> (queue out=w1238:refnum<queue>, error out=w1237:errorcluster)  [unwired: 1 in, 1 out]
          }
          frame #4 {
            n481 = for {
              N: 60 -> [w1251]
              i -> [w1250]
              n482 = Subtract(x=w1251, y=w1250) -> (x-y=w1249:i32)
              n483 = Decrement(x=w1249) -> (x-1=→"Low Cal\nCal Time Remain (sec)":i32)
              n484 = Wait (ms)(milliseconds to wait=u32 1000) -> ()  [unwired: 1 out]
            }
          }
          frame #5 {
            w1255 = FALSE
            n485 = Cluster To Array(cluster=T13 {"Message"="V2", "Message 3"="V4", "Message 4"="V1"}) -> (array=w1258:string[])
            n486 = for {
              tunnel: w1258 -> [w1265] mode=indexing
              tunnel: [w1264] -> w1254
              tunnel: [w1263] -> w1253
              tunnel: w1255 -> [w1262]
              tunnel: w1257 -> [w1261]
              tunnel: w1256 -> [w1260]
              n487 = Bundle(cluster=T4 {"Message"="", "Message Data"=variant} ("Message Cluster"), "Message"=w1265, "Message Data"=w1262) -> (w1267:T4)
              n488 = Enqueue Element(queue=w1261, element=w1267, error in (no error)=w1260) -> (queue out=w1264:refnum<queue>, error out=w1263:errorcluster)  [unwired: 1 in, 1 out]
            }
            n489 = local write "eV2"(w1255) -> ()
            n490 = local write "eV4"(w1255) -> ()
            n491 = local write "eV1"(w1255) -> ()
          }
          frame #6 {
            w1269 = 0.0 ("MFC_1\nSLPM Value")
            n492 = local write "MFC_1\nSLPM Value"(w1269) -> ()
            n493 = Bundle(cluster=T4 {"Message"="", "Message Data"=variant} ("Message Cluster"), "Message"="MFC_1", "Message Data"=w1269) -> (w1273:T4)
            n494 = Enqueue Element(queue=w1271, element=w1273, error in (no error)=w1270) -> (error out=w1268:errorcluster)  [unwired: 1 in, 2 out]
          }
          frame #7 {
            n495 = local write "Low Cal"(FALSE ("High Cal")) -> ()
          }
        }
      }
      event "Target Cal": Value Change {
        n496 = event-data() -> ()  [unwired: 1 in, 1 out]
        n497 = flat-sequence {
          tunnel: w1292 -> [w1300]
          tunnel: w1291 -> [w1299]
          tunnel: [w1298] -> w1290
          tunnel: [w1297] -> w1289
          tunnel: w1290 -> [w1306]
          tunnel: w1289 -> [w1305]
          tunnel: [w1303] -> w1287
          tunnel: [w1302] -> w1285
          tunnel: [w1311] -> w1288
          tunnel: w1287 -> [w1311]
          tunnel: [w1310] -> w1286
          tunnel: w1285 -> [w1310]
          tunnel: w1288 -> [w1321]
          tunnel: w1286 -> [w1320]
          tunnel: [w1318] -> w1283
          tunnel: [w1317] -> w1281
          tunnel: [w1327] -> w1284
          tunnel: w1283 -> [w1327]
          tunnel: [w1326] -> w1282
          tunnel: w1281 -> [w1326]
          tunnel: w1284 -> [w1336]
          tunnel: w1282 -> [w1335]
          tunnel: [w1333] -> w1280
          tunnel: [w1334] -> w1279
          tunnel: w1280 -> [w1351]
          tunnel: w1279 -> [w1350]
          tunnel: [w1348] -> w1277
          tunnel: [w1356] -> w1278
          tunnel: w1277 -> [w1356]
          frame #0 {
            w1296 = TRUE
            n498 = local write "eV4"(w1296) -> ()
            n499 = Bundle(cluster=T4 {"Message"="", "Message Data"=variant} ("Message Cluster"), "Message"="V4" ("Message 3"), "Message Data"=w1296) -> (w1295:T4)
            n500 = Enqueue Element(queue=w1300, element=w1295, error in (no error)=w1299) -> (queue out=w1298:refnum<queue>, error out=w1297:errorcluster)  [unwired: 1 in, 1 out]
          }
          frame #1 {
            n501 = local read "MFC_1 User Set Value"() -> (w1301:dbl)
            n502 = local write "MFC_1\nSLPM Value"(w1301) -> ()
            n503 = Bundle(cluster=T4 {"Message"="", "Message Data"=variant} ("Message Cluster"), "Message"="MFC_1", "Message Data"=w1301) -> (w1304:T4)
            n504 = Enqueue Element(queue=w1306, element=w1304, error in (no error)=w1305) -> (queue out=w1303:refnum<queue>, error out=w1302:errorcluster)  [unwired: 1 in, 1 out]
          }
          frame #2 {
            n505 = for {
              N: 45 -> [w1315]
              i -> [w1314]
              n506 = Subtract(x=w1315, y=w1314) -> (x-y=w1313:i32)
              n507 = Decrement(x=w1313) -> (x-1=→"Target Cal\nFlush Time Remain (sec)":i32)
              n508 = Wait (ms)(milliseconds to wait=u32 1000) -> ()  [unwired: 1 out]
            }
          }
          frame #3 {
            w1319 = TRUE
            n509 = Bundle(cluster=T4 {"Message"="", "Message Data"=variant} ("Message Cluster"), "Message"="V1", "Message Data"=w1319) -> (w1322:T4)
            n510 = local write "eV1"(w1319) -> ()
            n511 = Enqueue Element(queue=w1321, element=w1322, error in (no error)=w1320) -> (queue out=w1318:refnum<queue>, error out=w1317:errorcluster)  [unwired: 1 in, 1 out]
          }
          frame #4 {
            n512 = for {
              N: 60 -> [w1331]
              i -> [w1330]
              n513 = Subtract(x=w1331, y=w1330) -> (x-y=w1329:i32)
              n514 = Decrement(x=w1329) -> (x-1=→"Target Cal\nCal Time Remain (sec)":i32)
              n515 = Wait (ms)(milliseconds to wait=u32 1000) -> ()  [unwired: 1 out]
            }
          }
          frame #5 {
            w1339 = FALSE
            n516 = Cluster To Array(cluster=cluster{"Message 3":string, "Message":string} {"Message 3"="V4", "Message"="V1"}) -> (array=w1337:string[])
            n517 = for {
              tunnel: w1337 -> [w1345] mode=indexing
              tunnel: [w1344] -> w1333
              tunnel: [w1343] -> w1334
              tunnel: w1339 -> [w1342]
              tunnel: w1336 -> [w1341]
              tunnel: w1335 -> [w1340]
              n518 = Bundle(cluster=T4 {"Message"="", "Message Data"=variant} ("Message Cluster"), "Message"=w1345, "Message Data"=w1342) -> (w1347:T4)
              n519 = Enqueue Element(queue=w1341, element=w1347, error in (no error)=w1340) -> (queue out=w1344:refnum<queue>, error out=w1343:errorcluster)  [unwired: 1 in, 1 out]
            }
            n520 = local write "eV4"(w1339) -> ()
            n521 = local write "eV1"(w1339) -> ()
          }
          frame #6 {
            w1349 = 0.0 ("MFC_1\nSLPM Value")
            n522 = local write "MFC_1\nSLPM Value"(w1349) -> ()
            n523 = Bundle(cluster=T4 {"Message"="", "Message Data"=variant} ("Message Cluster"), "Message"="MFC_1", "Message Data"=w1349) -> (w1353:T4)
            n524 = Enqueue Element(queue=w1351, element=w1353, error in (no error)=w1350) -> (error out=w1348:errorcluster)  [unwired: 1 in, 2 out]
          }
          frame #7 {
            n525 = local write "Target Cal"(FALSE ("High Cal")) -> ()
          }
        }
      }
      event "MFC_1\nSLPM Value": Value Change {
        n526 = event-data() -> ()  [unwired: 1 in, 1 out]
        n527 = local read "MFC_1\nSLPM Value"() -> (w1357:dbl)
        n528 = Bundle(cluster=T4 {"Message"="", "Message Data"=variant} ("Message Cluster"), "Message"="MFC_1", "Message Data"=w1357) -> (w1361:T4)
        n529 = Enqueue Element(queue=w1360, element=w1361, error in (no error)=w1359) -> (error out=w1358:errorcluster)  [unwired: 1 in, 2 out]
      }
      event "FGGA UDP Time Offset": Value Change {
        n530 = event-data() -> ("NewVal"=w1364:i32)  [unwired: 1 in, 5 out]
        n531 = Bundle(cluster=T4 {"Message"="", "Message Data"=variant} ("Message Cluster"), "Message"="UDP Time Offset", "Message Data"=w1364) -> (w1368:T4)
        n532 = Enqueue Element(queue=w1367, element=w1368, error in (no error)=w1366) -> (error out=w1365:errorcluster)  [unwired: 1 in, 2 out]
      }
    }
    "FGGA Event Error out" <- w659
  }
  n533 = Create Network Stream Writer Endpoint(6:w53, 7:10 ("writer buffer size"), 9:w55, 10:"//192.168.101.17/command/reader/FGGA" ("reader url"), 11:"/command/writer/FGGA" ("writer name")) -> (0:w52:errorcluster, 3:w51:refnum<k21>)  [unwired: 2 in]
  n534 = node-c288(w11) -> ()  [unwired: 1 out]
  n535 = while {
    tunnel: w2 -> [w1378]
    shift-right: [w1373] -> _
    shift-left: w51 -> [w1375]
    shift-right: [w1371] -> w48
    shift-left: w52 -> [w1377]
    tunnel: w1 -> [w1372]
    stop <- w1371 stop-if-true
    # "FGGA UI Command Sender"
    n536 = Dequeue Element(queue=w1378, error in (no error)=w1372) -> (element=w1374:T4)  [unwired: 1 in, 3 out]
    n537 = Unbundle By Name(w1374) -> ("Message"=w1376:string)
    n538 = case shown="\"UDP Time Offset\"" w1376 {
      tunnel: w1377 -> [w1379 w1383 w1390 w1397 w1404 w1411 w1418 w1425 w1432 w1439 w1446]
      tunnel: w1375 -> [w1380 w1386 w1393 w1400 w1407 w1414 w1421 w1428 w1435 w1442 w1449]
      tunnel: w1374 -> [_ w1385 w1392 w1399 w1406 w1413 w1420 w1427 w1434 w1441 w1448]
      tunnel: [w1379 w1382 w1389 w1396 w1403 w1410 w1417 w1424 w1431 w1438 w1445] -> w1371
      tunnel: [w1380 w1381 w1388 w1395 w1402 w1409 w1416 w1423 w1430 w1437 w1444] -> w1373
      frame "False", Default {
      }
      frame "V1" {
        n539 = shared-variable-write(w1386, w1383, w1385) -> (w1384:refnum<k21>, w1387:errorcluster)  [unwired: 1 in, 1 out]
        n540 = Flush Stream(8:w1387, 11:w1384) -> (0:w1382:errorcluster, 3:w1381:refnum<k21>)  [unwired: 2 in, 1 out]
      }
      frame "MFC_1" {
        n541 = shared-variable-write(w1393, w1390, w1392) -> (w1391:refnum<k21>, w1394:errorcluster)  [unwired: 1 in, 1 out]
        n542 = Flush Stream(8:w1394, 11:w1391) -> (0:w1389:errorcluster, 3:w1388:refnum<k21>)  [unwired: 2 in, 1 out]
      }
      frame "UDP Time Offset" {
        n543 = shared-variable-write(w1400, w1397, w1399) -> (w1398:refnum<k21>, w1401:errorcluster)  [unwired: 1 in, 1 out]
        n544 = Flush Stream(8:w1401, 11:w1398) -> (0:w1396:errorcluster, 3:w1395:refnum<k21>)  [unwired: 2 in, 1 out]
      }
      frame "V2" {
        n545 = shared-variable-write(w1407, w1404, w1406) -> (w1405:refnum<k21>, w1408:errorcluster)  [unwired: 1 in, 1 out]
        n546 = Flush Stream(8:w1408, 11:w1405) -> (0:w1403:errorcluster, 3:w1402:refnum<k21>)  [unwired: 2 in, 1 out]
      }
      frame "V3" {
        n547 = shared-variable-write(w1414, w1411, w1413) -> (w1412:refnum<k21>, w1415:errorcluster)  [unwired: 1 in, 1 out]
        n548 = Flush Stream(8:w1415, 11:w1412) -> (0:w1410:errorcluster, 3:w1409:refnum<k21>)  [unwired: 2 in, 1 out]
      }
      frame "V4" {
        n549 = shared-variable-write(w1421, w1418, w1420) -> (w1419:refnum<k21>, w1422:errorcluster)  [unwired: 1 in, 1 out]
        n550 = Flush Stream(8:w1422, 11:w1419) -> (0:w1417:errorcluster, 3:w1416:refnum<k21>)  [unwired: 2 in, 1 out]
      }
      frame "FGGA_pump" {
        n551 = shared-variable-write(w1428, w1425, w1427) -> (w1426:refnum<k21>, w1429:errorcluster)  [unwired: 1 in, 1 out]
        n552 = Flush Stream(8:w1429, 11:w1426) -> (0:w1424:errorcluster, 3:w1423:refnum<k21>)  [unwired: 2 in, 1 out]
      }
      frame "Flight Number" {
        n553 = shared-variable-write(w1435, w1432, w1434) -> (w1433:refnum<k21>, w1436:errorcluster)  [unwired: 1 in, 1 out]
        n554 = Flush Stream(8:w1436, 11:w1433) -> (0:w1431:errorcluster, 3:w1430:refnum<k21>)  [unwired: 2 in, 1 out]
      }
      frame "FGGA_restart" {
        n555 = shared-variable-write(w1442, w1439, w1441) -> (w1440:refnum<k21>, w1443:errorcluster)  [unwired: 1 in, 1 out]
        n556 = Flush Stream(8:w1443, 11:w1440) -> (0:w1438:errorcluster, 3:w1437:refnum<k21>)  [unwired: 2 in, 1 out]
      }
      frame "Stop File Write" {
        n557 = shared-variable-write(w1449, w1446, w1448) -> (w1447:refnum<k21>, w1450:errorcluster)  [unwired: 1 in, 1 out]
        n558 = Flush Stream(8:w1450, 11:w1447) -> (0:w1445:errorcluster, 3:w1444:refnum<k21>)  [unwired: 2 in, 1 out]
      }
    }
  }
  "FGGA command sender error out" <- w48
  n559 = Obtain Queue(name (unnamed)="SO2_Command", element data type=w37) -> (queue out=w46:refnum<queue>, error out=w39:errorcluster)  [unwired: 3 in, 1 out]
  n560 = while {
    tunnel: w46 -> [w1454]
    tunnel: w39 -> [w1453]
    tunnel: [w1451] -> _
    stop <- FALSE stop-if-true
    # "SO2 UI Event Handler Loop"
    n561 = event shown="[1] \"SO2 Flush\": Value Change" {
      selector: _ -> [_ _ _ _ _ _ _ _ _ _ _ _ _ _ _ _ _ _]
      dyn-events: _ -> [_ _ _ _ _ _ _ _ _ _ _ _ _ _ _ _ _ _]
      timeout: _ -> [_ _ _ _ _ _ _ _ _ _ _ _ _ _ _ _ _ _]
      tunnel: w1454 -> [w1461 w1473 w1522 w1561 w1630 w1637 w1641 w1648 w1655 w1662 w1669 w1676 w1683 w1690 w1697 w1704 w1711 w1718]
      tunnel: w1453 -> [w1460 w1472 w1521 w1560 w1629 w1636 w1640 w1647 w1654 w1661 w1668 w1675 w1682 w1689 w1696 w1703 w1710 w1717]
      tunnel: [w1455 w1471 w1520 _ w1624 w1631 w1639 w1646 w1653 w1660 w1667 w1674 w1681 w1688 w1695 w1702 w1709 w1716] -> w1451
      event "eV9": Value Change {
        n562 = event-data() -> ("NewVal"=w1458:bool)  [unwired: 1 in]
        n563 = Bundle(cluster=T4 {"Message"="", "Message Data"=variant} ("Message Cluster"), "Message"="V9", "Message Data"=w1458) -> (w1456:T4)
        n564 = Enqueue Element(queue=w1461, element=w1456, error in (no error)=w1460) -> (error out=w1455:errorcluster)  [unwired: 1 in, 2 out]
      }
      event "SO2 Flush": Value Change {
        n565 = event-data() -> ()  [unwired: 1 in, 1 out]
        n566 = flat-sequence {
          tunnel: w1473 -> [w1481]
          tunnel: w1472 -> [w1480]
          tunnel: [w1476] -> w1468
          tunnel: [w1474] -> w1466
          tunnel: w1468 -> [w1483]
          tunnel: [w1485] -> w1467
          tunnel: w1466 -> [w1484]
          tunnel: [w1486] -> w1465
          tunnel: w1467 -> [w1492]
          tunnel: [w1492] -> w1470
          tunnel: [w1490] -> w1469
          tunnel: w1465 -> [w1490]
          tunnel: w1470 -> [w1501]
          tunnel: [w1500] -> w1464
          tunnel: w1469 -> [w1502]
          tunnel: [w1498] -> w1462
          tunnel: w1464 -> [w1508]
          tunnel: [w1509] -> w1463
          tunnel: w1462 -> [w1507]
          tunnel: [w1514] -> w1471
          tunnel: w1463 -> [w1514]
          frame #0 {
            w1475 = TRUE ("SO2 Flush")
            n567 = Bundle(cluster=T4 {"Message"="", "Message Data"=variant} ("Message Cluster"), "Message"="V9", "Message Data"=w1475) -> (w1477:T4)
            n568 = local write "eV9"(w1475) -> ()
            n569 = Enqueue Element(queue=w1481, element=w1477, error in (no error)=w1480) -> (queue out=w1474:refnum<queue>, error out=w1476:errorcluster)  [unwired: 1 in, 1 out]
          }
          frame #1 {
            n570 = local read "MFC_2 User Set Value"() -> (w1482:dbl)
            n571 = local write "MFC_2\nSLPM Value"(w1482) -> ()
            n572 = Bundle(cluster=T4 {"Message"="", "Message Data"=variant} ("Message Cluster"), "Message"="MFC_2", "Message Data"=w1482) -> (w1487:T4)
            n573 = Enqueue Element(queue=w1484, element=w1487, error in (no error)=w1483) -> (queue out=w1486:refnum<queue>, error out=w1485:errorcluster)  [unwired: 1 in, 1 out]
          }
          frame #2 {
            n574 = for {
              N: "eV9 Flush User\nset time (sec)" -> [w1496]
              i -> [w1495]
              n575 = Subtract(x=w1496, y=w1495) -> (x-y=w1494:i32)
              n576 = Decrement(x=w1494) -> (x-1=w1493:i32)
              n577 = local write "SO2 Flush\nTime Remain (sec)"(w1493) -> ()
              n578 = Wait (ms)(milliseconds to wait=u32 1000) -> ()  [unwired: 1 out]
            }
          }
          frame #3 {
            w1499 = FALSE
            n579 = Bundle(cluster=T4 {"Message"="", "Message Data"=variant} ("Message Cluster"), "Message"="V9", "Message Data"=w1499) -> (w1503:T4)
            n580 = local write "eV9"(w1499) -> ()
            n581 = Enqueue Element(queue=w1502, element=w1503, error in (no error)=w1501) -> (queue out=w1498:refnum<queue>, error out=w1500:errorcluster)  [unwired: 1 in, 1 out]
          }
          frame #4 {
            w1506 = 0.0 ("MFC_2\nSLPM Value")
            n582 = local write "MFC_2\nSLPM Value"(w1506) -> ()
            n583 = Bundle(cluster=T4 {"Message"="", "Message Data"=variant} ("Message Cluster"), "Message"="MFC_2", "Message Data"=w1506) -> (w1510:T4)
            n584 = Enqueue Element(queue=w1507, element=w1510, error in (no error)=w1508) -> (error out=w1509:errorcluster)  [unwired: 1 in, 2 out]
          }
          frame #5 {
            n585 = local write "SO2 Flush"(FALSE ("SO2 Flush")) -> ()
          }
        }
      }
      event "SO2 Zeroing": Value Change {
        n586 = event-data() -> ()  [unwired: 1 in, 1 out]
        n587 = flat-sequence {
          tunnel: w1522 -> [w1530]
          tunnel: w1521 -> [w1529]
          tunnel: [w1525] -> w1519
          tunnel: [w1523] -> w1515
          tunnel: w1519 -> [w1533]
          tunnel: [w1533] -> w1518
          tunnel: [w1531] -> w1516
          tunnel: w1515 -> [w1531]
          tunnel: w1518 -> [w1541]
          tunnel: [w1540] -> w1517
          tunnel: w1516 -> [w1542]
          tunnel: [w1547] -> w1520
          tunnel: w1517 -> [w1547]
          frame #0 {
            w1524 = TRUE ("SO2 Flush")
            n588 = local write "SO2 eV6"(w1524) -> ()
            n589 = Bundle(cluster=T4 {"Message"="", "Message Data"=variant} ("Message Cluster"), "Message"="V6", "Message Data"=w1524) -> (w1526:T4)
            n590 = Enqueue Element(queue=w1530, element=w1526, error in (no error)=w1529) -> (queue out=w1523:refnum<queue>, error out=w1525:errorcluster)  [unwired: 1 in, 1 out]
          }
          frame #1 {
            # "10 Mins Count down"
            n591 = for {
              N: 600 -> [w1537]
              i -> [w1536]
              n592 = Subtract(x=w1537, y=w1536) -> (x-y=w1535:i32)
              n593 = Decrement(x=w1535) -> (x-1=w1534:i32)
              n594 = local write "SO2 Zeroing\nTime Remain (sec)"(w1534) -> ()
              n595 = Wait (ms)(milliseconds to wait=u32 1000) -> ()  [unwired: 1 out]
            }
          }
          frame #2 {
            w1539 = FALSE
            n596 = Bundle(cluster=T4 {"Message"="", "Message Data"=variant} ("Message Cluster"), "Message"="V6", "Message Data"=w1539) -> (w1543:T4)
            n597 = local write "SO2 eV6"(w1539) -> ()
            n598 = Enqueue Element(queue=w1542, element=w1543, error in (no error)=w1541) -> (error out=w1540:errorcluster)  [unwired: 1 in, 2 out]
          }
          frame #3 {
            n599 = local write "SO2 Zeroing"(FALSE ("SO2 Flush")) -> ()
          }
        }
      }
      event "SO2 CAL": Value Change {
        n600 = event-data() -> ()  [unwired: 1 in, 1 out]
        n601 = flat-sequence {
          tunnel: w1561 -> [w1569]
          tunnel: w1560 -> [w1568]
          tunnel: [w1564] -> w1559
          tunnel: [w1563] -> w1557
          tunnel: w1559 -> [w1573]
          tunnel: [w1572] -> w1558
          tunnel: w1557 -> [w1574]
          tunnel: [w1570] -> w1555
          tunnel: w1558 -> [w1580]
          tunnel: [w1580] -> w1556
          tunnel: w1555 -> [w1578]
          tunnel: [w1578] -> w1554
          tunnel: w1556 -> [w1589]
          tunnel: w1554 -> [w1590]
          tunnel: [w1587] -> w1552
          tunnel: [w1586] -> w1550
          tunnel: [w1595] -> w1553
          tunnel: w1552 -> [w1595]
          tunnel: [w1594] -> w1551
          tunnel: w1550 -> [w1594]
          tunnel: w1553 -> [w1605]
          tunnel: w1551 -> [w1604]
          tunnel: [w1603] -> w1549
          tunnel: [w1602] -> w1548
          tunnel: w1549 -> [w1619]
          tunnel: w1548 -> [w1618]
          frame #0 {
            w1562 = TRUE ("SO2 Flush")
            n602 = Bundle(cluster=T4 {"Message"="", "Message Data"=variant} ("Message Cluster"), "Message"="V9", "Message Data"=w1562) -> (w1565:T4)
            n603 = local write "eV9"(w1562) -> ()
            n604 = Enqueue Element(queue=w1569, element=w1565, error in (no error)=w1568) -> (queue out=w1563:refnum<queue>, error out=w1564:errorcluster)  [unwired: 1 in, 1 out]
          }
          frame #1 {
            n605 = local read "MFC_2 User Set Value"() -> (w1571:dbl)
            n606 = local write "MFC_2\nSLPM Value"(w1571) -> ()
            n607 = Bundle(cluster=T4 {"Message"="", "Message Data"=variant} ("Message Cluster"), "Message"="MFC_2", "Message Data"=w1571) -> (w1575:T4)
            n608 = Enqueue Element(queue=w1574, element=w1575, error in (no error)=w1573) -> (queue out=w1570:refnum<queue>, error out=w1572:errorcluster)  [unwired: 1 in, 1 out]
          }
          frame #2 {
            n609 = for {
              N: "eV9 flush User\nset time (sec)" -> [w1584]
              i -> [w1583]
              n610 = Subtract(x=w1584, y=w1583) -> (x-y=w1582:i32)
              n611 = Decrement(x=w1582) -> (x-1=w1581:i32)
              n612 = local write "SO2 Flush\nTime Remain (sec)"(w1581) -> ()
              n613 = Wait (ms)(milliseconds to wait=u32 1000) -> ()  [unwired: 1 out]
            }
          }
          frame #3 {
            w1588 = TRUE ("SO2 Flush")
            n614 = Bundle(cluster=T4 {"Message"="", "Message Data"=variant} ("Message Cluster"), "Message"="V8", "Message Data"=w1588) -> (w1591:T4)
            n615 = local write "eV8"(w1588) -> ()
            n616 = Enqueue Element(queue=w1590, element=w1591, error in (no error)=w1589) -> (queue out=w1587:refnum<queue>, error out=w1586:errorcluster)  [unwired: 1 in, 1 out]
          }
          frame #4 {
            n617 = for {
              N: "eV8 User\nset time (sec)" -> [w1600]
              i -> [w1599]
              n618 = Subtract(x=w1600, y=w1599) -> (x-y=w1598:i32)
              n619 = Decrement(x=w1598) -> (x-1=w1597:i32)
              n620 = local write "SO2 CAL\nTime Remain (sec)"(w1597) -> ()
              n621 = Wait (ms)(milliseconds to wait=u32 1000) -> ()  [unwired: 1 out]
            }
          }
          frame #5 {
            n622 = Cluster To Array(cluster=cluster{"Message":string, "Message 2":string} {"Message"="V8", "Message 2"="V9"}) -> (array=w1607:string[])
            n623 = for {
              tunnel: w1607 -> [w1614] mode=indexing
              tunnel: FALSE ("SO2 Flush") -> [w1613]
              tunnel: w1605 -> [w1612]
              tunnel: w1604 -> [w1611]
              tunnel: [w1610] -> w1603
              tunnel: [w1609] -> w1602
              n624 = Bundle(cluster=T4 {"Message"="", "Message Data"=variant} ("Message Cluster"), "Message"=w1614, "Message Data"=w1613) -> (w1615:T4)
              n625 = Enqueue Element(queue=w1612, element=w1615, error in (no error)=w1611) -> (queue out=w1610:refnum<queue>, error out=w1609:errorcluster)  [unwired: 1 in, 1 out]
            }
          }
          frame #6 {
            w1617 = 0.0 ("MFC_2\nSLPM Value")
            n626 = local write "MFC_2\nSLPM Value"(w1617) -> ()
            n627 = Bundle(cluster=T4 {"Message"="", "Message Data"=variant} ("Message Cluster"), "Message"="MFC_2", "Message Data"=w1617) -> (w1620:T4)
            n628 = Enqueue Element(queue=w1619, element=w1620, error in (no error)=w1618) -> ()  [unwired: 1 in, 3 out]
          }
          frame #7 {
            w1623 = FALSE ("SO2 Flush")
            n629 = local write "SO2 CAL"(w1623) -> ()
            n630 = local write "eV9"(w1623) -> ()
            n631 = local write "eV8"(w1623) -> ()
          }
        }
      }
      event "MFC_2\nSLPM Value": Value Change {
        n632 = event-data() -> ("NewVal"=w1627:dbl)  [unwired: 1 in]
        n633 = Bundle(cluster=T4 {"Message"="", "Message Data"=variant} ("Message Cluster"), "Message"="MFC_2", "Message Data"=w1627) -> (w1625:T4)
        n634 = Enqueue Element(queue=w1630, element=w1625, error in (no error)=w1629) -> (error out=w1624:errorcluster)  [unwired: 1 in, 2 out]
      }
      event "MFC_3\nSLPM Value": Value Change {
        n635 = event-data() -> ("NewVal"=w1634:dbl)  [unwired: 1 in]
        n636 = Bundle(cluster=T4 {"Message"="", "Message Data"=variant} ("Message Cluster"), "Message"="MFC_3", "Message Data"=w1634) -> (w1632:T4)
        n637 = Enqueue Element(queue=w1637, element=w1632, error in (no error)=w1636) -> (error out=w1631:errorcluster)  [unwired: 1 in, 2 out]
      }
      event "eV8": Value Change {
        n638 = event-data() -> ("NewVal"=w1638:bool)  [unwired: 1 in]
        n639 = Bundle(cluster=T4 {"Message"="", "Message Data"=variant} ("Message Cluster"), "Message"="V8", "Message Data"=w1638) -> (w1642:T4)
        n640 = Enqueue Element(queue=w1641, element=w1642, error in (no error)=w1640) -> (error out=w1639:errorcluster)  [unwired: 1 in, 2 out]
      }
      event "SO2 eV6": Value Change {
        n641 = event-data() -> ("NewVal"=w1645:bool)  [unwired: 1 in]
        n642 = Bundle(cluster=T4 {"Message"="", "Message Data"=variant} ("Message Cluster"), "Message"="V6", "Message Data"=w1645) -> (w1649:T4)
        n643 = Enqueue Element(queue=w1648, element=w1649, error in (no error)=w1647) -> (error out=w1646:errorcluster)  [unwired: 1 in, 2 out]
      }
      event "Simulate Conc": Value Change {
        n644 = event-data() -> ("NewVal"=w1652:bool)  [unwired: 1 in]
        n645 = Bundle(cluster=T4 {"Message"="", "Message Data"=variant} ("Message Cluster"), "Message"="Simulate Conc", "Message Data"=w1652) -> (w1656:T4)
        n646 = Enqueue Element(queue=w1655, element=w1656, error in (no error)=w1654) -> (error out=w1653:errorcluster)  [unwired: 1 in, 2 out]
      }
      event "SO2 UDP Time Offset": Value Change {
        n647 = event-data() -> ("NewVal"=w1659:i32)  [unwired: 1 in]
        n648 = Bundle(cluster=T4 {"Message"="", "Message Data"=variant} ("Message Cluster"), "Message"="UDP Time Offset", "Message Data"=w1659) -> (w1663:T4)
        n649 = Enqueue Element(queue=w1662, element=w1663, error in (no error)=w1661) -> (error out=w1660:errorcluster)  [unwired: 1 in, 2 out]
      }
      event "Simulate STEL Conc": Value Change {
        n650 = event-data() -> ("NewVal"=w1666:dbl)  [unwired: 1 in]
        n651 = Bundle(cluster=T4 {"Message"="", "Message Data"=variant} ("Message Cluster"), "Message"="Simulate STEL Conc", "Message Data"=w1666) -> (w1670:T4)
        n652 = Enqueue Element(queue=w1669, element=w1670, error in (no error)=w1668) -> (error out=w1667:errorcluster)  [unwired: 1 in, 2 out]
      }
      event "Simulate TWA Conc": Value Change {
        n653 = event-data() -> ("NewVal"=w1673:dbl)  [unwired: 1 in]
        n654 = Bundle(cluster=T4 {"Message"="", "Message Data"=variant} ("Message Cluster"), "Message"="Simulate TWA Conc", "Message Data"=w1673) -> (w1677:T4)
        n655 = Enqueue Element(queue=w1676, element=w1677, error in (no error)=w1675) -> (error out=w1674:errorcluster)  [unwired: 1 in, 2 out]
      }
      event "10mins STEL Limit": Value Change {
        n656 = event-data() -> ("NewVal"=w1680:i32)  [unwired: 1 in]
        n657 = Bundle(cluster=T4 {"Message"="", "Message Data"=variant} ("Message Cluster"), "Message"="10mins STEL Limit", "Message Data"=w1680) -> (w1684:T4)
        n658 = Enqueue Element(queue=w1683, element=w1684, error in (no error)=w1682) -> (error out=w1681:errorcluster)  [unwired: 1 in, 2 out]
      }
      event "8hr TWA Limit": Value Change {
        n659 = event-data() -> ("NewVal"=w1687:i32)  [unwired: 1 in]
        n660 = Bundle(cluster=T4 {"Message"="", "Message Data"=variant} ("Message Cluster"), "Message"="8hr TWA Limit", "Message Data"=w1687) -> (w1691:T4)
        n661 = Enqueue Element(queue=w1690, element=w1691, error in (no error)=w1689) -> (error out=w1688:errorcluster)  [unwired: 1 in, 2 out]
      }
      event "SO2 Offset": Value Change {
        n662 = event-data() -> ("NewVal"=w1694:dbl)  [unwired: 1 in]
        n663 = Bundle(cluster=T4 {"Message"="", "Message Data"=variant} ("Message Cluster"), "Message"="Offset", "Message Data"=w1694) -> (w1698:T4)
        n664 = Enqueue Element(queue=w1697, element=w1698, error in (no error)=w1696) -> (error out=w1695:errorcluster)  [unwired: 1 in, 2 out]
      }
      event "SO2 Slope": Value Change {
        n665 = event-data() -> ("NewVal"=w1701:dbl)  [unwired: 1 in]
        n666 = Bundle(cluster=T4 {"Message"="", "Message Data"=variant} ("Message Cluster"), "Message"="Slope", "Message Data"=w1701) -> (w1705:T4)
        n667 = Enqueue Element(queue=w1704, element=w1705, error in (no error)=w1703) -> (error out=w1702:errorcluster)  [unwired: 1 in, 2 out]
      }
      event "Confirm Flight Number": Value Change {
        n668 = event-data() -> ()  [unwired: 1 in, 6 out]
        n669 = local read "Flight Number"() -> (w1708:string)
        n670 = Bundle(cluster=T4 {"Message"="", "Message Data"=variant} ("Message Cluster"), "Message"="Flight Number", "Message Data"=w1708) -> (w1712:T4)
        n671 = Enqueue Element(queue=w1711, element=w1712, error in (no error)=w1710) -> (error out=w1709:errorcluster)  [unwired: 1 in, 2 out]
      }
      event "cRIO File IO Stop\n(USB Flash Drive Unmount)": Value Change {
        n672 = event-data() -> ("NewVal"=w1715:bool)  [unwired: 1 in]
        n673 = Bundle(cluster=T4 {"Message"="", "Message Data"=variant} ("Message Cluster"), "Message"="Stop File Write", "Message Data"=w1715) -> (w1719:T4)
        n674 = Enqueue Element(queue=w1718, element=w1719, error in (no error)=w1717) -> (error out=w1716:errorcluster)  [unwired: 1 in, 2 out]
      }
    }
    "SO2 Event error out" <- w1451
  }
  n675 = Create Network Stream Writer Endpoint(6:w43, 7:10 ("writer buffer size"), 9:w37, 10:"//192.168.101.17/command/reader/SO2" ("reader url"), 11:"/command/writer/SO2" ("writer name")) -> (0:w42:errorcluster, 3:w41:refnum<k21>)  [unwired: 2 in]
  n676 = while {
    tunnel: w46 -> [w1729]
    shift-right: [w1724] -> _
    shift-left: w41 -> [w1726]
    shift-right: [w1722] -> w38
    shift-left: w42 -> [w1728]
    tunnel: w39 -> [w1723]
    stop <- w1722 stop-if-true
    # "SO2 UI Command Sender"
    n677 = Dequeue Element(queue=w1729, error in (no error)=w1723) -> (element=w1725:T4)  [unwired: 1 in, 3 out]
    n678 = Unbundle By Name(w1725) -> ("Message"=w1727:string)
    n679 = case shown="\"UDP Time Offset\"" w1727 {
      tunnel: w1728 -> [w1730 w1734 w1741 w1748 w1755 w1762 w1769 w1776 w1783 w1790 w1797 w1804 w1811 w1818 w1825 w1832]
      tunnel: w1726 -> [w1731 w1737 w1744 w1751 w1758 w1765 w1772 w1779 w1786 w1793 w1800 w1807 w1814 w1821 w1828 w1835]
      tunnel: w1725 -> [_ w1736 w1743 w1750 w1757 w1764 w1771 w1778 w1785 w1792 w1799 w1806 w1813 w1820 w1827 w1834]
      tunnel: [w1730 w1733 w1740 w1747 w1754 w1761 w1768 w1775 w1782 w1789 w1796 w1803 w1810 w1817 w1824 w1831] -> w1722
      tunnel: [w1731 w1732 w1739 w1746 w1753 w1760 w1767 w1774 w1781 w1788 w1795 w1802 w1809 w1816 w1823 w1830] -> w1724
      frame "False", Default {
      }
      frame "V9" {
        n680 = shared-variable-write(w1737, w1734, w1736) -> (w1735:refnum<k21>, w1738:errorcluster)  [unwired: 1 in, 1 out]
        n681 = Flush Stream(8:w1738, 11:w1735) -> (0:w1733:errorcluster, 3:w1732:refnum<k21>)  [unwired: 2 in, 1 out]
      }
      frame "MFC_2" {
        n682 = shared-variable-write(w1744, w1741, w1743) -> (w1742:refnum<k21>, w1745:errorcluster)  [unwired: 1 in, 1 out]
        n683 = Flush Stream(8:w1745, 11:w1742) -> (0:w1740:errorcluster, 3:w1739:refnum<k21>)  [unwired: 2 in, 1 out]
      }
      frame "MFC_3" {
        n684 = shared-variable-write(w1751, w1748, w1750) -> (w1749:refnum<k21>, w1752:errorcluster)  [unwired: 1 in, 1 out]
        n685 = Flush Stream(8:w1752, 11:w1749) -> (0:w1747:errorcluster, 3:w1746:refnum<k21>)  [unwired: 2 in, 1 out]
      }
      frame "V6" {
        n686 = shared-variable-write(w1758, w1755, w1757) -> (w1756:refnum<k21>, w1759:errorcluster)  [unwired: 1 in, 1 out]
        n687 = Flush Stream(8:w1759, 11:w1756) -> (0:w1754:errorcluster, 3:w1753:refnum<k21>)  [unwired: 2 in, 1 out]
      }
      frame "Simulate Conc" {
        n688 = shared-variable-write(w1765, w1762, w1764) -> (w1763:refnum<k21>, w1766:errorcluster)  [unwired: 1 in, 1 out]
        n689 = Flush Stream(8:w1766, 11:w1763) -> (0:w1761:errorcluster, 3:w1760:refnum<k21>)  [unwired: 2 in, 1 out]
      }
      frame "Simulate STEL Conc" {
        n690 = shared-variable-write(w1772, w1769, w1771) -> (w1770:refnum<k21>, w1773:errorcluster)  [unwired: 1 in, 1 out]
        n691 = Flush Stream(8:w1773, 11:w1770) -> (0:w1768:errorcluster, 3:w1767:refnum<k21>)  [unwired: 2 in, 1 out]
      }
      frame "Simulate TWA Conc" {
        n692 = shared-variable-write(w1779, w1776, w1778) -> (w1777:refnum<k21>, w1780:errorcluster)  [unwired: 1 in, 1 out]
        n693 = Flush Stream(8:w1780, 11:w1777) -> (0:w1775:errorcluster, 3:w1774:refnum<k21>)  [unwired: 2 in, 1 out]
      }
      frame "10mins STEL Limit" {
        n694 = shared-variable-write(w1786, w1783, w1785) -> (w1784:refnum<k21>, w1787:errorcluster)  [unwired: 1 in, 1 out]
        n695 = Flush Stream(8:w1787, 11:w1784) -> (0:w1782:errorcluster, 3:w1781:refnum<k21>)  [unwired: 2 in, 1 out]
      }
      frame "8hr TWA Limit" {
        n696 = shared-variable-write(w1793, w1790, w1792) -> (w1791:refnum<k21>, w1794:errorcluster)  [unwired: 1 in, 1 out]
        n697 = Flush Stream(8:w1794, 11:w1791) -> (0:w1789:errorcluster, 3:w1788:refnum<k21>)  [unwired: 2 in, 1 out]
      }
      frame "Offset" {
        n698 = shared-variable-write(w1800, w1797, w1799) -> (w1798:refnum<k21>, w1801:errorcluster)  [unwired: 1 in, 1 out]
        n699 = Flush Stream(8:w1801, 11:w1798) -> (0:w1796:errorcluster, 3:w1795:refnum<k21>)  [unwired: 2 in, 1 out]
      }
      frame "Slope" {
        n700 = shared-variable-write(w1807, w1804, w1806) -> (w1805:refnum<k21>, w1808:errorcluster)  [unwired: 1 in, 1 out]
        n701 = Flush Stream(8:w1808, 11:w1805) -> (0:w1803:errorcluster, 3:w1802:refnum<k21>)  [unwired: 2 in, 1 out]
      }
      frame "Flight Number" {
        n702 = shared-variable-write(w1814, w1811, w1813) -> (w1812:refnum<k21>, w1815:errorcluster)  [unwired: 1 in, 1 out]
        n703 = Flush Stream(8:w1815, 11:w1812) -> (0:w1810:errorcluster, 3:w1809:refnum<k21>)  [unwired: 2 in, 1 out]
      }
      frame "Stop File Write" {
        n704 = shared-variable-write(w1821, w1818, w1820) -> (w1819:refnum<k21>, w1822:errorcluster)  [unwired: 1 in, 1 out]
        n705 = Flush Stream(8:w1822, 11:w1819) -> (0:w1817:errorcluster, 3:w1816:refnum<k21>)  [unwired: 2 in, 1 out]
      }
      frame "UDP Time Offset" {
        n706 = shared-variable-write(w1828, w1825, w1827) -> (w1826:refnum<k21>, w1829:errorcluster)  [unwired: 1 in, 1 out]
        n707 = Flush Stream(8:w1829, 11:w1826) -> (0:w1824:errorcluster, 3:w1823:refnum<k21>)  [unwired: 2 in, 1 out]
      }
      frame "V8" {
        n708 = shared-variable-write(w1835, w1832, w1834) -> (w1833:refnum<k21>, w1836:errorcluster)  [unwired: 1 in, 1 out]
        n709 = Flush Stream(8:w1836, 11:w1833) -> (0:w1831:errorcluster, 3:w1830:refnum<k21>)  [unwired: 2 in, 1 out]
      }
    }
  }
  "SO2 command sender error out" <- w38
  n710 = Obtain Queue(name (unnamed)="TEi43c_Command", element data type=w26) -> (queue out=w35:refnum<queue>, error out=w28:errorcluster)  [unwired: 3 in, 1 out]
  n711 = Create Network Stream Writer Endpoint(6:w32, 7:10 ("writer buffer size"), 9:w26, 10:"//192.168.101.17/command/reader/TEi43c" ("reader url"), 11:"/command/writer/TEi43c" ("writer name")) -> (0:w31:errorcluster, 3:w30:refnum<k21>)  [unwired: 2 in]
  n712 = while {
    tunnel: w35 -> [w1840]
    tunnel: w28 -> [w1839]
    tunnel: [w1837] -> _
    stop <- FALSE stop-if-true
    # "TEi43c Ozone UI Event Handler Loop"
    n713 = event shown="[0] \"Ozone Zeroing\": Value Change" {
      selector: _ -> [_ _ _ _ _]
      dyn-events: _ -> [_ _ _ _ _]
      timeout: _ -> [_ _ _ _ _]
      tunnel: w1840 -> [w1848 w1876 w1884 w1891 w1898]
      tunnel: w1839 -> [w1847 w1875 w1883 w1890 w1897]
      tunnel: [w1846 w1874 w1882 w1889 w1896] -> w1837
      event "Ozone Zeroing": Value Change {
        n714 = event-data() -> ()  [unwired: 1 in, 6 out]
        n715 = flat-sequence {
          tunnel: w1848 -> [w1853]
          tunnel: w1847 -> [w1852]
          tunnel: [w1851] -> w1845
          tunnel: [w1849] -> w1841
          tunnel: w1845 -> [w1859]
          tunnel: [w1859] -> w1844
          tunnel: [w1857] -> w1842
          tunnel: w1841 -> [w1857]
          tunnel: w1844 -> [w1867]
          tunnel: [w1866] -> w1843
          tunnel: w1842 -> [w1868]
          tunnel: [w1873] -> w1846
          tunnel: w1843 -> [w1873]
          frame #0 {
            w1850 = TRUE
            n716 = local write "Ozone eV6"(w1850) -> ()
            n717 = Bundle(cluster=T4 {"Message"="", "Message Data"=variant} ("Message Cluster"), "Message"="V6", "Message Data"=w1850) -> (w1854:T4)
            n718 = Enqueue Element(queue=w1853, element=w1854, error in (no error)=w1852) -> (queue out=w1849:refnum<queue>, error out=w1851:errorcluster)  [unwired: 1 in, 1 out]
          }
          frame #1 {
            # "10 Mins Count down"
            n719 = for {
              N: 600 -> [w1863]
              i -> [w1862]
              n720 = Subtract(x=w1863, y=w1862) -> (x-y=w1861:i32)
              n721 = Decrement(x=w1861) -> (x-1=→"Ozone Zeroing\nTime Remain (sec)":i32)
              n722 = Wait (ms)(milliseconds to wait=u32 1000) -> ()  [unwired: 1 out]
            }
          }
          frame #2 {
            w1865 = FALSE
            n723 = local write "Ozone eV6"(w1865) -> ()
            n724 = Bundle(cluster=T4 {"Message"="", "Message Data"=variant} ("Message Cluster"), "Message"="V6", "Message Data"=w1865) -> (w1869:T4)
            n725 = Enqueue Element(queue=w1868, element=w1869, error in (no error)=w1867) -> (error out=w1866:errorcluster)  [unwired: 1 in, 2 out]
          }
          frame #3 {
            n726 = local write "Ozone Zeroing"(FALSE ("Ozone Zeroing")) -> ()
          }
        }
      }
      event "Ozone eV6": Value Change {
        n727 = event-data() -> ("NewVal"=w1877:bool)  [unwired: 1 in]
        n728 = Bundle(cluster=T4 {"Message"="", "Message Data"=variant} ("Message Cluster"), "Message"="V6", "Message Data"=w1877) -> (w1878:T4)
        n729 = Enqueue Element(queue=w1876, element=w1878, error in (no error)=w1875) -> (error out=w1874:errorcluster)  [unwired: 1 in, 2 out]
      }
      event "cRIO File IO Stop\n(USB Flash Drive Unmount)": Value Change {
        n730 = event-data() -> ("NewVal"=w1881:bool)  [unwired: 1 in]
        n731 = Bundle(cluster=T4 {"Message"="", "Message Data"=variant} ("Message Cluster"), "Message"="Stop File Write", "Message Data"=w1881) -> (w1885:T4)
        n732 = Enqueue Element(queue=w1884, element=w1885, error in (no error)=w1883) -> (error out=w1882:errorcluster)  [unwired: 1 in, 2 out]
      }
      event "Ozone UDP Time Offset": Value Change {
        n733 = event-data() -> ("NewVal"=w1888:i32)  [unwired: 1 in]
        n734 = Bundle(cluster=T4 {"Message"="", "Message Data"=variant} ("Message Cluster"), "Message"="UDP Time Offset", "Message Data"=w1888) -> (w1892:T4)
        n735 = Enqueue Element(queue=w1891, element=w1892, error in (no error)=w1890) -> (error out=w1889:errorcluster)  [unwired: 1 in, 2 out]
      }
      event "Confirm Flight Number": Value Change {
        n736 = event-data() -> ()  [unwired: 1 in, 5 out]
        n737 = local read "Flight Number"() -> (w1895:string)
        n738 = Bundle(cluster=T4 {"Message"="", "Message Data"=variant} ("Message Cluster"), "Message"="Flight Number", "Message Data"=w1895) -> (w1899:T4)
        n739 = Enqueue Element(queue=w1898, element=w1899, error in (no error)=w1897) -> (error out=w1896:errorcluster)  [unwired: 1 in, 2 out]
      }
    }
    "Ozone Event error out" <- w1837
  }
  n740 = while {
    tunnel: w35 -> [w1909]
    shift-right: [w1904] -> _
    shift-left: w30 -> [w1906]
    shift-right: [w1902] -> w27
    shift-left: w31 -> [w1908]
    tunnel: w28 -> [w1903]
    stop <- w1902 stop-if-true
    # "TEi43c Ozone UI Command Sender"
    n741 = Dequeue Element(queue=w1909, error in (no error)=w1903) -> (element=w1905:T4)  [unwired: 1 in, 3 out]
    n742 = Unbundle By Name(w1905) -> ("Message"=w1907:string)
    n743 = case shown="\"UDP Time Offset\"" w1907 {
      tunnel: w1908 -> [w1910 w1914 w1921 w1928 w1935]
      tunnel: w1906 -> [w1911 w1917 w1924 w1931 w1938]
      tunnel: w1905 -> [_ w1916 w1923 w1930 w1937]
      tunnel: [w1910 w1913 w1920 w1927 w1934] -> w1902
      tunnel: [w1911 w1912 w1919 w1926 w1933] -> w1904
      frame "False", Default {
      }
      frame "V6" {
        n744 = shared-variable-write(w1917, w1914, w1916) -> (w1915:refnum<k21>, w1918:errorcluster)  [unwired: 1 in, 1 out]
        n745 = Flush Stream(8:w1918, 11:w1915) -> (0:w1913:errorcluster, 3:w1912:refnum<k21>)  [unwired: 2 in, 1 out]
      }
      frame "Stop File Write" {
        n746 = shared-variable-write(w1924, w1921, w1923) -> (w1922:refnum<k21>, w1925:errorcluster)  [unwired: 1 in, 1 out]
        n747 = Flush Stream(8:w1925, 11:w1922) -> (0:w1920:errorcluster, 3:w1919:refnum<k21>)  [unwired: 2 in, 1 out]
      }
      frame "Flight Number" {
        n748 = shared-variable-write(w1931, w1928, w1930) -> (w1929:refnum<k21>, w1932:errorcluster)  [unwired: 1 in, 1 out]
        n749 = Flush Stream(8:w1932, 11:w1929) -> (0:w1927:errorcluster, 3:w1926:refnum<k21>)  [unwired: 2 in, 1 out]
      }
      frame "UDP Time Offset" {
        n750 = shared-variable-write(w1938, w1935, w1937) -> (w1936:refnum<k21>, w1939:errorcluster)  [unwired: 1 in, 1 out]
        n751 = Flush Stream(8:w1939, 11:w1936) -> (0:w1934:errorcluster, 3:w1933:refnum<k21>)  [unwired: 2 in, 1 out]
      }
    }
  }
  "Ozone command sender error out" <- w27
  n752 = Obtain Queue(name (unnamed)="2BOzone_Command", element data type=w14) -> (queue out=w23:refnum<queue>, error out=w16:errorcluster)  [unwired: 3 in, 1 out]
  n753 = Create Network Stream Writer Endpoint(6:w20, 7:10 ("writer buffer size"), 9:w14, 10:"//192.168.101.17/command/reader/2BOzone" ("reader url"), 11:"/command/writer/2BOzone" ("writer name")) -> (0:w19:errorcluster, 3:w18:refnum<k21>)  [unwired: 2 in]
  n754 = while {
    tunnel: w23 -> [w1943]
    tunnel: w16 -> [w1942]
    tunnel: [w1940] -> _
    stop <- FALSE stop-if-true
    # "2BOzone UI Event Handler Loop"
    n755 = event shown="[7] \"Confirm Flight Number\": Value Change" {
      selector: _ -> [_ _ _ _ _ _ _ _]
      dyn-events: _ -> [_ _ _ _ _ _ _ _]
      timeout: _ -> [_ _ _ _ _ _ _ _]
      tunnel: w1943 -> [w1947 w1954 w1961 w1968 w1975 w1982 w1989 w1996]
      tunnel: w1942 -> [w1946 w1953 w1960 w1967 w1974 w1981 w1988 w1995]
      tunnel: [w1945 w1952 w1959 w1966 w1973 w1980 w1987 w1994] -> w1940
      event "Ambient = OFF\nCabin = ON": Value Change {
        n756 = event-data() -> ("NewVal"=w1944:bool)  [unwired: 1 in]
        n757 = Bundle(cluster=T4 {"Message"="", "Message Data"=variant} ("Message Cluster"), "Message"="Ambient/Cabin", "Message Data"=w1944) -> (w1948:T4)
        n758 = Enqueue Element(queue=w1947, element=w1948, error in (no error)=w1946) -> (error out=w1945:errorcluster)  [unwired: 1 in, 2 out]
      }
      event "Simulate 2B Conc": Value Change {
        n759 = event-data() -> ("NewVal"=w1951:bool)  [unwired: 1 in]
        n760 = Bundle(cluster=T4 {"Message"="", "Message Data"=variant} ("Message Cluster"), "Message"="Simulate_conc", "Message Data"=w1951) -> (w1955:T4)
        n761 = Enqueue Element(queue=w1954, element=w1955, error in (no error)=w1953) -> (error out=w1952:errorcluster)  [unwired: 1 in, 2 out]
      }
      event "Simulate Inst Conc": Value Change {
        n762 = event-data() -> ("NewVal"=w1958:i32)  [unwired: 1 in]
        n763 = Bundle(cluster=T4 {"Message"="", "Message Data"=variant} ("Message Cluster"), "Message"="Simulate_inst_conc", "Message Data"=w1958) -> (w1962:T4)
        n764 = Enqueue Element(queue=w1961, element=w1962, error in (no error)=w1960) -> (error out=w1959:errorcluster)  [unwired: 1 in, 2 out]
      }
      event "Inst_alm_thresh": Value Change {
        n765 = event-data() -> ("NewVal"=w1965:i32)  [unwired: 1 in]
        n766 = Bundle(cluster=T4 {"Message"="", "Message Data"=variant} ("Message Cluster"), "Message"="Inst_alm_thresh", "Message Data"=w1965) -> (w1969:T4)
        n767 = Enqueue Element(queue=w1968, element=w1969, error in (no error)=w1967) -> (error out=w1966:errorcluster)  [unwired: 1 in, 2 out]
      }
      event "3hr_alm_thresh": Value Change {
        n768 = event-data() -> ("NewVal"=w1972:i32)  [unwired: 1 in]
        n769 = Bundle(cluster=T4 {"Message"="", "Message Data"=variant} ("Message Cluster"), "Message"="3hr_alm_thresh", "Message Data"=w1972) -> (w1976:T4)
        n770 = Enqueue Element(queue=w1975, element=w1976, error in (no error)=w1974) -> (error out=w1973:errorcluster)  [unwired: 1 in, 2 out]
      }
      event "Simulate 3hr Average Conc": Value Change {
        n771 = event-data() -> ("NewVal"=w1979:dbl)  [unwired: 1 in]
        n772 = Bundle(cluster=T4 {"Message"="", "Message Data"=variant} ("Message Cluster"), "Message"="Simulate_3hr_av_conc", "Message Data"=w1979) -> (w1983:T4)
        n773 = Enqueue Element(queue=w1982, element=w1983, error in (no error)=w1981) -> (error out=w1980:errorcluster)  [unwired: 1 in, 2 out]
      }
      event "cRIO File IO Stop\n(USB Flash Drive Unmount)": Value Change {
        n774 = event-data() -> ("NewVal"=w1986:bool)  [unwired: 1 in]
        n775 = Bundle(cluster=T4 {"Message"="", "Message Data"=variant} ("Message Cluster"), "Message"="Stop File Write", "Message Data"=w1986) -> (w1990:T4)
        n776 = Enqueue Element(queue=w1989, element=w1990, error in (no error)=w1988) -> (error out=w1987:errorcluster)  [unwired: 1 in, 2 out]
      }
      event "Confirm Flight Number": Value Change {
        n777 = event-data() -> ()  [unwired: 1 in, 5 out]
        n778 = local read "Flight Number"() -> (w1993:string)
        n779 = Bundle(cluster=T4 {"Message"="", "Message Data"=variant} ("Message Cluster"), "Message"="Flight Number", "Message Data"=w1993) -> (w1997:T4)
        n780 = Enqueue Element(queue=w1996, element=w1997, error in (no error)=w1995) -> (error out=w1994:errorcluster)  [unwired: 1 in, 2 out]
      }
    }
    "2BOzone Event error out" <- w1940
  }
  n781 = while {
    tunnel: w23 -> [w2007]
    shift-right: [w2002] -> _
    shift-left: w18 -> [w2004]
    shift-right: [w2000] -> w15
    shift-left: w19 -> [w2006]
    tunnel: w16 -> [w2001]
    stop <- w2000 stop-if-true
    # "2BOzone UI Command Sender"
    n782 = Dequeue Element(queue=w2007, error in (no error)=w2001) -> (element=w2003:T4)  [unwired: 1 in, 3 out]
    n783 = Unbundle By Name(w2003) -> ("Message"=w2005:string)
    n784 = case shown="\"3hr_alm_thresh\"" w2005 {
      tunnel: w2006 -> [w2008 w2012 w2019 w2026 w2033 w2040 w2047 w2054 w2061]
      tunnel: w2004 -> [w2009 w2015 w2022 w2029 w2036 w2043 w2050 w2057 w2064]
      tunnel: w2003 -> [_ w2014 w2021 w2028 w2035 w2042 w2049 w2056 w2063]
      tunnel: [w2008 w2011 w2018 w2025 w2032 w2039 w2046 w2053 w2060] -> w2000
      tunnel: [w2009 w2010 w2017 w2024 w2031 w2038 w2045 w2052 w2059] -> w2002
      frame "False", Default {
      }
      frame "Ambient/Cabin" {
        n785 = shared-variable-write(w2015, w2012, w2014) -> (w2013:refnum<k21>, w2016:errorcluster)  [unwired: 1 in, 1 out]
        n786 = Flush Stream(8:w2016, 11:w2013) -> (0:w2011:errorcluster, 3:w2010:refnum<k21>)  [unwired: 2 in, 1 out]
      }
      frame "Simulate_conc" {
        n787 = shared-variable-write(w2022, w2019, w2021) -> (w2020:refnum<k21>, w2023:errorcluster)  [unwired: 1 in, 1 out]
        n788 = Flush Stream(8:w2023, 11:w2020) -> (0:w2018:errorcluster, 3:w2017:refnum<k21>)  [unwired: 2 in, 1 out]
      }
      frame "Simulate_inst_conc" {
        n789 = shared-variable-write(w2029, w2026, w2028) -> (w2027:refnum<k21>, w2030:errorcluster)  [unwired: 1 in, 1 out]
        n790 = Flush Stream(8:w2030, 11:w2027) -> (0:w2025:errorcluster, 3:w2024:refnum<k21>)  [unwired: 2 in, 1 out]
      }
      frame "Inst_alm_thresh" {
        n791 = shared-variable-write(w2036, w2033, w2035) -> (w2034:refnum<k21>, w2037:errorcluster)  [unwired: 1 in, 1 out]
        n792 = Flush Stream(8:w2037, 11:w2034) -> (0:w2032:errorcluster, 3:w2031:refnum<k21>)  [unwired: 2 in, 1 out]
      }
      frame "3hr_alm_thresh" {
        n793 = shared-variable-write(w2043, w2040, w2042) -> (w2041:refnum<k21>, w2044:errorcluster)  [unwired: 1 in, 1 out]
        n794 = Flush Stream(8:w2044, 11:w2041) -> (0:w2039:errorcluster, 3:w2038:refnum<k21>)  [unwired: 2 in, 1 out]
      }
      frame "Simulate_3hr_av_conc" {
        n795 = shared-variable-write(w2050, w2047, w2049) -> (w2048:refnum<k21>, w2051:errorcluster)  [unwired: 1 in, 1 out]
        n796 = Flush Stream(8:w2051, 11:w2048) -> (0:w2046:errorcluster, 3:w2045:refnum<k21>)  [unwired: 2 in, 1 out]
      }
      frame "Stop File Write" {
        n797 = shared-variable-write(w2057, w2054, w2056) -> (w2055:refnum<k21>, w2058:errorcluster)  [unwired: 1 in, 1 out]
        n798 = Flush Stream(8:w2058, 11:w2055) -> (0:w2053:errorcluster, 3:w2052:refnum<k21>)  [unwired: 2 in, 1 out]
      }
      frame "Flight Number" {
        n799 = shared-variable-write(w2064, w2061, w2063) -> (w2062:refnum<k21>, w2065:errorcluster)  [unwired: 1 in, 1 out]
        n800 = Flush Stream(8:w2065, 11:w2062) -> (0:w2060:errorcluster, 3:w2059:refnum<k21>)  [unwired: 2 in, 1 out]
      }
    }
  }
  "2BOzone command sender error out" <- w15
